vi "Main.vi"() -> ()   [LabVIEW 2020, in "Ex 1 - Simulated LP.lvlib"]
uses:
  Ex 1 - Simulated LP.lvlib
  <vilib>/measure/macond.llb/IIR Filter for 1 Chan.vi
  <vilib>/measure/matone.llb/Extract Single Tone Information 1 Chan.vi
  <vilib>/measure/NI_MABase.lvlib
  <vilib>/measure/NI_MAPro.lvlib
panel:
  in  "Title":string="BODE PLOT (FH Joanneum)"
  in  "Cut-off Frequency":dbl=100000.0 format="%#_6p"
  in  "Order":i32=2
  in  "Topology":T1(ring)=enum."Butterworth"
  in  "Start":bool
  in  "Timing (ms)":u32
  in  "stop":bool
  in  "Amplitude":dbl=10.0
  in  "Freq. Step":dbl=1000.0 caption="Frequency Step" format="%#_6p"
  in  "Stop Frequ.":dbl=1000000.0 caption="Stop Frequency" format="%#_6p"
  in  "Start Freq.":dbl=1000.0 caption="Start Frequency" format="%#_6p"
  out "Waveform Graph":waveform(dbl)[](graph)
  out "Magnitude":cluster{"X":dbl, "Y":dbl}[](graph)=[{"X"=1000.0, "Y"=0.0}, {"X"=2000.0, "Y"=0.0}, {"X"=3000.0, "Y"=-4.7058926481545906e-07}, {"X"=4000.0, "Y"=-4.235994406084898e-06}, {"X"=5000.0, "Y"=-1.5203059229301419e-05}, {"X"=6000.0, "Y"=-3.8126734506028564e-05}, {"X"=7000.0, "Y"=-7.876650446461324e-05}, {"X"=8000.0, "Y"=-0.0001439147572122518}, {"X"=9000.0, "Y"=-0.00024140357010209228}, {"X"=10000.0, "Y"=-0.00038010648213580877}, {"X"=11000.0, "Y"=-0.0005699385936490564}, {"X"=12000.0, "Y"=-0.0008218558292255898}, {"X"=13000.0, "Y"=-0.0011478535749765322}, {"X"=14000.0, "Y"=-0.001560964706777549}, {"X"=15000.0, "Y"=-0.0020752569545813126}, {"X"=16000.0, "Y"=-0.0027058295134445385}, {"X"=17000.0, "Y"=-0.003468808794544552}, {"X"=18000.0, "Y"=-0.004381343195914282}, {"X"=19000.0, "Y"=-0.005461596762600354}, {"X"=20000.0, "Y"=-0.006728741598133291}, {"X"=21000.0, "Y"=-0.008202948881267663}, {"X"=22000.0, "Y"=-0.009905378335483283}, {"X"=23000.0, "Y"=-0.011858165993133746}, {"X"=24000.0, "Y"=-0.01408441009127886}, {"X"=25000.0, "Y"=-0.016608154932204067}, {"X"=26000.0, "Y"=-0.019454372539159805}, {"X"=27000.0, "Y"=-0.022648941935728285}, {"X"=28000.0, "Y"=-0.026218625878250468}, {"X"=29000.0, "Y"=-0.030191044870233313}, {"X"=30000.0, "Y"=-0.03459464829307458}, {"X"=31000.0, "Y"=-0.0394586824895382}, {"X"=32000.0, "Y"=-0.04481315564715423}, {"X"=33000.0, "Y"=-0.05068879933203461}, {"X"=34000.0, "Y"=-0.05711702654319666}, {"X"=35000.0, "Y"=-0.06412988616203336}, {"X"=36000.0, "Y"=-0.07176001369565913}, {"X"=37000.0, "Y"=-0.0800405782282296}, {"X"=38000.0, "Y"=-0.08900522551567218}, {"X"=39000.0, "Y"=-0.09868801718765945}, {"X"=40000.0, "Y"=-0.10912336604225487}, {"X"=41000.0, "Y"=-0.12034596745431009}, {"X"=42000.0, "Y"=-0.1323907269484053}, {"X"=43000.0, "Y"=-0.14529268402125897}, {"X"=44000.0, "Y"=-0.15908693233963056}, {"X"=45000.0, "Y"=-0.1738085364745352}, {"X"=46000.0, "Y"=-0.18949244537640458}, {"X"=47000.0, "Y"=-0.20617340283688407}, {"X"=48000.0, "Y"=-0.223885855226176}, {"X"=49000.0, "Y"=-0.24266385683539424}, {"X"=50000.0, "Y"=-0.26254097319813513}, {"X"=51000.0, "Y"=-0.2835501828093141}, {"X"=52000.0, "Y"=-0.305723777689094}, {"X"=53000.0, "Y"=-0.3290932632891572}, {"X"=54000.0, "Y"=-0.3536892700554042}, {"X"=55000.0, "Y"=-0.37954141196215424}, {"X"=56000.0, "Y"=-0.4066782422305516}, {"X"=57000.0, "Y"=-0.4351271247729583}, {"X"=58000.0, "Y"=-0.46491414587534396}, {"X"=59000.0, "Y"=-0.49606402204891537}, {"X"=60000.0, "Y"=-0.5286000113418585}, {"X"=61000.0, "Y"=-0.5625438287314889}, {"X"=62000.0, "Y"=-0.5979155661973111}, {"X"=63000.0, "Y"=-0.6347336180540024}, {"X"=64000.0, "Y"=-0.6730146121003455}, {"X"=65000.0, "Y"=-0.7127733470961873}, {"X"=66000.0, "Y"=-0.7540227370395547}, {"X"=67000.0, "Y"=-0.7967737626708788}, {"X"=68000.0, "Y"=-0.8410354305647758}, {"X"=69000.0, "Y"=-0.8868147401211939}, {"X"=70000.0, "Y"=-0.9341166586949998}, {"X"=71000.0, "Y"=-0.9829441050379926}, {"X"=72000.0, "Y"=-1.0332979411576286}, {"X"=73000.0, "Y"=-1.085176972621999}, {"X"=74000.0, "Y"=-1.1385779572743775}, {"X"=75000.0, "Y"=-1.1934956222444086}, {"X"=76000.0, "Y"=-1.2499226890777513}, {"X"=77000.0, "Y"=-1.307849906737507}, {"X"=78000.0, "Y"=-1.367266092175559}, {"X"=79000.0, "Y"=-1.4281581781011314}, {"X"=80000.0, "Y"=-1.490511267540837}, {"X"=81000.0, "Y"=-1.5543086947183857}, {"X"=82000.0, "Y"=-1.619532091760238}, {"X"=83000.0, "Y"=-1.6861614606881672}, {"X"=84000.0, "Y"=-1.7541752501398347}, {"X"=85000.0, "Y"=-1.8235504362403714}, {"X"=86000.0, "Y"=-1.894262607028815}, {"X"=87000.0, "Y"=-1.9662860498489467}, {"X"=88000.0, "Y"=-2.039593841103528}, {"X"=89000.0, "Y"=-2.1141579377887303}, {"X"=90000.0, "Y"=-2.189949270229024}, {"X"=91000.0, "Y"=-2.2669378354594665}, {"X"=92000.0, "Y"=-2.345092790717058}, {"X"=93000.0, "Y"=-2.424382546535789}, {"X"=94000.0, "Y"=-2.504774858965561}, {"X"=95000.0, "Y"=-2.586236920475759}, {"X"=96000.0, "Y"=-2.668735449101548}, {"X"=97000.0, "Y"=-2.752236775525848}, {"X"=98000.0, "Y"=-2.8367069276892405}, {"X"=99000.0, "Y"=-2.922111712666817}, {"X"=100000.0, "Y"=-3.008416795542534}, {"X"=101000.0, "Y"=-3.0955877750590197}, {"X"=102000.0, "Y"=-3.18359025585552}, {"X"=103000.0, "Y"=-3.272389917143707}, {"X"=104000.0, "Y"=-3.3619525777045487}, {"X"=105000.0, "Y"=-3.452244257121428}, {"X"=106000.0, "Y"=-3.5432312331963423}, {"X"=107000.0, "Y"=-3.634880095522957}, {"X"=108000.0, "Y"=-3.7271577952177553}, {"X"=109000.0, "Y"=-3.820031690834062}, {"X"=110000.0, "Y"=-3.913469590505059}, {"X"=111000.0, "Y"=-4.007439790382403}, {"X"=112000.0, "Y"=-4.101911109452055}, {"X"=113000.0, "Y"=-4.196852920828556}, {"X"=114000.0, "Y"=-4.292235179634819}, {"X"=115000.0, "Y"=-4.3880284475928875}, {"X"=116000.0, "Y"=-4.484203914453854}, {"X"=117000.0, "Y"=-4.580733416407038}, {"X"=118000.0, "Y"=-4.677589451610474}, {"X"=119000.0, "Y"=-4.774745192989594}, {"X"=120000.0, "Y"=-4.872174498456132}, {"X"=121000.0, "Y"=-4.96985191869544}, {"X"=122000.0, "Y"=-5.067752702673315}, {"X"=123000.0, "Y"=-5.165855460663462}, {"X"=124000.0, "Y"=-5.2641319673999405}, {"X"=125000.0, "Y"=-5.362561822358578}, {"X"=126000.0, "Y"=-5.461123081246283}, {"X"=127000.0, "Y"=-5.5597944964429304}, {"X"=128000.0, "Y"=-5.658555511891694}, {"X"=129000.0, "Y"=-5.757386256696502}, {"X"=130000.0, "Y"=-5.8562675375405355}, {"X"=131000.0, "Y"=-5.955180830049295}, {"X"=132000.0, "Y"=-6.0541082692101345}, {"X"=133000.0, "Y"=-6.1530326389465}, {"X"=134000.0, "Y"=-6.251937360956765}, {"X"=135000.0, "Y"=-6.3508064829043125}, {"X"=136000.0, "Y"=-6.449624666050838}, {"X"=137000.0, "Y"=-6.548377172415963}, {"X"=138000.0, "Y"=-6.64704985153692}, {"X"=139000.0, "Y"=-6.745629126905376}, {"X"=140000.0, "Y"=-6.844101982144563}, {"X"=141000.0, "Y"=-6.942455946989798}, {"X"=142000.0, "Y"=-7.040679083126048}, {"X"=143000.0, "Y"=-7.138759969940191}, {"X"=144000.0, "Y"=-7.236687690232017}, {"X"=145000.0, "Y"=-7.334451815927893}, {"X"=146000.0, "Y"=-7.432042393834642}, {"X"=147000.0, "Y"=-7.529449931475854}, {"X"=148000.0, "Y"=-7.626665383033114}, {"X"=149000.0, "Y"=-7.723680135429653}, {"X"=150000.0, "Y"=-7.820485994576546}, {"X"=151000.0, "Y"=-7.917075171808563}, {"X"=152000.0, "Y"=-8.013440270519457}, {"X"=153000.0, "Y"=-8.109574273030688}, {"X"=154000.0, "Y"=-8.205470527694786}, {"X"=155000.0, "Y"=-8.301122736248846}, {"X"=156000.0, "Y"=-8.39652494143235}, {"X"=157000.0, "Y"=-8.491671514879934}, {"X"=158000.0, "Y"=-8.586557145285052}, {"X"=159000.0, "Y"=-8.681176826856413}, {"X"=160000.0, "Y"=-8.775525848057779}, {"X"=161000.0, "Y"=-8.869599780639252}, {"X"=162000.0, "Y"=-8.963394468965031}, {"X"=163000.0, "Y"=-9.05690601963175}, {"X"=164000.0, "Y"=-9.150130791383427}, {"X"=165000.0, "Y"=-9.24306538531414}, {"X"=166000.0, "Y"=-9.335706635368732}, {"X"=167000.0, "Y"=-9.42805159912396}, {"X"=168000.0, "Y"=-9.520097548858109}, {"X"=169000.0, "Y"=-9.611841962904887}, {"X"=170000.0, "Y"=-9.703282517275158}, {"X"=171000.0, "Y"=-9.794417077563297}, {"X"=172000.0, "Y"=-9.885243691108869}, {"X"=173000.0, "Y"=-9.975760579431988}, {"X"=174000.0, "Y"=-10.065966130914283}, {"X"=175000.0, "Y"=-10.155858893742307}, {"X"=176000.0, "Y"=-10.245437569088836}, {"X"=177000.0, "Y"=-10.334701004534255}, {"X"=178000.0, "Y"=-10.423648187726064}, {"X"=179000.0, "Y"=-10.512278240262589}, {"X"=180000.0, "Y"=-10.600590411796667}, {"X"=181000.0, "Y"=-10.688584074359479}, {"X"=182000.0, "Y"=-10.776258716886478}, {"X"=183000.0, "Y"=-10.863613939954625}, {"X"=184000.0, "Y"=-10.950649450707068}, {"X"=185000.0, "Y"=-11.037365057981665}, {"X"=186000.0, "Y"=-11.123760667607058}, {"X"=187000.0, "Y"=-11.209836277898013}, {"X"=188000.0, "Y"=-11.295591975305555}, {"X"=189000.0, "Y"=-11.381027930247125}, {"X"=190000.0, "Y"=-11.466144393097576}, {"X"=191000.0, "Y"=-11.55094169032801}, {"X"=192000.0, "Y"=-11.635420220809047}, {"X"=193000.0, "Y"=-11.719580452252224}, {"X"=194000.0, "Y"=-11.803422917791085}, {"X"=195000.0, "Y"=-11.886948212708035}, {"X"=196000.0, "Y"=-11.970156991279863}, {"X"=197000.0, "Y"=-12.053049963763204}, {"X"=198000.0, "Y"=-12.135627893489993}, {"X"=199000.0, "Y"=-12.217891594089759}, {"X"=200000.0, "Y"=-12.29984192682171}, {"X"=201000.0, "Y"=-12.381479798015718}, {"X"=202000.0, "Y"=-12.46280615661728}, {"X"=203000.0, "Y"=-12.543821991840698}, {"X"=204000.0, "Y"=-12.62452833091158}, {"X"=205000.0, "Y"=-12.70492623690393}, {"X"=206000.0, "Y"=-12.78501680667606}, {"X"=207000.0, "Y"=-12.864801168882458}, {"X"=208000.0, "Y"=-12.944280482076318}, {"X"=209000.0, "Y"=-13.023455932887927}, {"X"=210000.0, "Y"=-13.102328734286502}, {"X"=211000.0, "Y"=-13.180900123907104}, {"X"=212000.0, "Y"=-13.25917136245713}, {"X"=213000.0, "Y"=-13.337143732188219}, {"X"=214000.0, "Y"=-13.414818535431191}, {"X"=215000.0, "Y"=-13.492197093200705}, {"X"=216000.0, "Y"=-13.569280743854248}, {"X"=217000.0, "Y"=-13.646070841812053}, {"X"=218000.0, "Y"=-13.72256875633643}, {"X"=219000.0, "Y"=-13.798775870356472}, {"X"=220000.0, "Y"=-13.8746935793548}, {"X"=221000.0, "Y"=-13.950323290295861}, {"X"=222000.0, "Y"=-14.025666420605168}, {"X"=223000.0, "Y"=-14.100724397194575}, {"X"=224000.0, "Y"=-14.17549865552884}, {"X"=225000.0, "Y"=-14.24999063874024}, {"X"=226000.0, "Y"=-14.324201796771556}, {"X"=227000.0, "Y"=-14.398133585574461}, {"X"=228000.0, "Y"=-14.471787466329765}, {"X"=229000.0, "Y"=-14.545164904715811}, {"X"=230000.0, "Y"=-14.618267370197653}, {"X"=231000.0, "Y"=-14.691096335362255}, {"X"=232000.0, "Y"=-14.763653275275736}, {"X"=233000.0, "Y"=-14.835939666878035}, {"X"=234000.0, "Y"=-14.907956988400237}, {"X"=235000.0, "Y"=-14.979706718812793}, {"X"=236000.0, "Y"=-15.05119033729854}, {"X"=237000.0, "Y"=-15.122409322755534}, {"X"=238000.0, "Y"=-15.193365153317533}, {"X"=239000.0, "Y"=-15.264059305905214}, {"X"=240000.0, "Y"=-15.334493255794165}, {"X"=241000.0, "Y"=-15.404668476206185}, {"X"=242000.0, "Y"=-15.474586437922506}, {"X"=243000.0, "Y"=-15.544248608915323}, {"X"=244000.0, "Y"=-15.61365645399822}, {"X"=245000.0, "Y"=-15.682811434497662}, {"X"=246000.0, "Y"=-15.751715007934507}, {"X"=247000.0, "Y"=-15.820368627733375}, {"X"=248000.0, "Y"=-15.888773742935978}, {"X"=249000.0, "Y"=-15.956931797937868}, {"X"=250000.0, "Y"=-16.024844232238152}, {"X"=251000.0, "Y"=-16.0925124802025}, {"X"=252000.0, "Y"=-16.15993797083511}, {"X"=253000.0, "Y"=-16.227122127574578}, {"X"=254000.0, "Y"=-16.294066368090544}, {"X"=255000.0, "Y"=-16.360772104096878}, {"X"=256000.0, "Y"=-16.42724074118115}, {"X"=257000.0, "Y"=-16.493473678633453}, {"X"=258000.0, "Y"=-16.559472309295167}, {"X"=259000.0, "Y"=-16.625238019415402}, {"X"=260000.0, "Y"=-16.690772188512703}, {"X"=261000.0, "Y"=-16.756076189253196}, {"X"=262000.0, "Y"=-16.82115138732697}, {"X"=263000.0, "Y"=-16.885999141346083}, {"X"=264000.0, "Y"=-16.950620802738797}, {"X"=265000.0, "Y"=-17.015017715654785}, {"X"=266000.0, "Y"=-17.079191216883608}, {"X"=267000.0, "Y"=-17.143142635769106}, {"X"=268000.0, "Y"=-17.206873294141282}, {"X"=269000.0, "Y"=-17.270384506246447}, {"X"=270000.0, "Y"=-17.33367757868715}, {"X"=271000.0, "Y"=-17.396753810367407}, {"X"=272000.0, "Y"=-17.45961449244436}, {"X"=273000.0, "Y"=-17.522260908281318}, {"X"=274000.0, "Y"=-17.58469433341141}, {"X"=275000.0, "Y"=-17.646916035498602}, {"X"=276000.0, "Y"=-17.708927274314817}, {"X"=277000.0, "Y"=-17.770729301707398}, {"X"=278000.0, "Y"=-17.832323361580443}, {"X"=279000.0, "Y"=-17.893710689877405}, {"X"=280000.0, "Y"=-17.954892514566296}, {"X"=281000.0, "Y"=-18.01587005563178}, {"X"=282000.0, "Y"=-18.07664452506634}, {"X"=283000.0, "Y"=-18.137217126865238}, {"X"=284000.0, "Y"=-18.197589057027997}, {"X"=285000.0, "Y"=-18.257761503562023}, {"X"=286000.0, "Y"=-18.31773564648534}, {"X"=287000.0, "Y"=-18.377512657836736}, {"X"=288000.0, "Y"=-18.43709370168274}, {"X"=289000.0, "Y"=-18.496479934135166}, {"X"=290000.0, "Y"=-18.555672503361244}, {"X"=291000.0, "Y"=-18.614672549604855}, {"X"=292000.0, "Y"=-18.673481205205256}, {"X"=293000.0, "Y"=-18.73209959461389}, {"X"=294000.0, "Y"=-18.79052883442349}, {"X"=295000.0, "Y"=-18.848770033390608}, {"X"=296000.0, "Y"=-18.90682429245923}, {"X"=297000.0, "Y"=-18.964692704793407}, {"X"=298000.0, "Y"=-19.02237635580446}, {"X"=299000.0, "Y"=-19.079876323179942}, {"X"=300000.0, "Y"=-19.137193676920692}, {"X"=301000.0, "Y"=-19.194329479368367}, {"X"=302000.0, "Y"=-19.25128478524589}, {"X"=303000.0, "Y"=-19.30806064168852}, {"X"=304000.0, "Y"=-19.36465808828178}, {"X"=305000.0, "Y"=-19.42107815710046}, {"X"=306000.0, "Y"=-19.477321872746593}, {"X"=307000.0, "Y"=-19.533390252386738}, {"X"=308000.0, "Y"=-19.589284305794557}, {"X"=309000.0, "Y"=-19.645005035390913}, {"X"=310000.0, "Y"=-19.70055343628699}, {"X"=311000.0, "Y"=-19.75593049632279}, {"X"=312000.0, "Y"=-19.811137196111925}, {"X"=313000.0, "Y"=-19.86617450908731}, {"X"=314000.0, "Y"=-19.921043401540246}, {"X"=315000.0, "Y"=-19.975744832667978}, {"X"=316000.0, "Y"=-20.03027975461794}, {"X"=317000.0, "Y"=-20.084649112531817}, {"X"=318000.0, "Y"=-20.13885384459283}, {"X"=319000.0, "Y"=-20.192894882068188}, {"X"=320000.0, "Y"=-20.24677314935738}, {"X"=321000.0, "Y"=-20.30048956403927}, {"X"=322000.0, "Y"=-20.35404503691563}, {"X"=323000.0, "Y"=-20.407440472061595}, {"X"=324000.0, "Y"=-20.46067676686917}, {"X"=325000.0, "Y"=-20.513754812092763}, {"X"=326000.0, "Y"=-20.566675491902643}, {"X"=327000.0, "Y"=-20.619439683925968}, {"X"=328000.0, "Y"=-20.672048259297352}, {"X"=329000.0, "Y"=-20.724502082703424}, {"X"=330000.0, "Y"=-20.77680201243293}, {"X"=331000.0, "Y"=-20.828948900420343}, {"X"=332000.0, "Y"=-20.880943592297548}, {"X"=333000.0, "Y"=-20.932786927438933}, {"X"=334000.0, "Y"=-20.9844797390068}, {"X"=335000.0, "Y"=-21.036022853999793}, {"X"=336000.0, "Y"=-21.08741709330269}, {"X"=337000.0, "Y"=-21.138663271728486}, {"X"=338000.0, "Y"=-21.189762198067818}, {"X"=339000.0, "Y"=-21.240714675137014}, {"X"=340000.0, "Y"=-21.29152149982074}, {"X"=341000.0, "Y"=-21.342183463123405}, {"X"=342000.0, "Y"=-21.392701350207087}, {"X"=343000.0, "Y"=-21.44307594045021}, {"X"=344000.0, "Y"=-21.493308007482206}, {"X"=345000.0, "Y"=-21.543398319233695}, {"X"=346000.0, "Y"=-21.59334763798313}, {"X"=347000.0, "Y"=-21.643156720399933}, {"X"=348000.0, "Y"=-21.692826317589663}, {"X"=349000.0, "Y"=-21.742357175140654}, {"X"=350000.0, "Y"=-21.791750033167908}, {"X"=351000.0, "Y"=-21.84100562635718}, {"X"=352000.0, "Y"=-21.89012468401001}, {"X"=353000.0, "Y"=-21.939107930083615}, {"X"=354000.0, "Y"=-21.987956083242338}, {"X"=355000.0, "Y"=-22.036669856894306}, {"X"=356000.0, "Y"=-22.085249959237782}, {"X"=357000.0, "Y"=-22.133697093305603}, {"X"=358000.0, "Y"=-22.18201195700206}, {"X"=359000.0, "Y"=-22.23019524314994}, {"X"=360000.0, "Y"=-22.278247639534484}, {"X"=361000.0, "Y"=-22.326169828940024}, {"X"=362000.0, "Y"=-22.37396248919461}, {"X"=363000.0, "Y"=-22.42162629321072}, {"X"=364000.0, "Y"=-22.46916190902627}, {"X"=365000.0, "Y"=-22.51656999984677}, {"X"=366000.0, "Y"=-22.563851224082892}, {"X"=367000.0, "Y"=-22.61100623539201}, {"X"=368000.0, "Y"=-22.658035682721156}, {"X"=369000.0, "Y"=-22.70494021034019}, {"X"=370000.0, "Y"=-22.751720457886616}, {"X"=371000.0, "Y"=-22.798377060403567}, {"X"=372000.0, "Y"=-22.844910648375144}, {"X"=373000.0, "Y"=-22.89132184776854}, {"X"=374000.0, "Y"=-22.93761128007275}, {"X"=375000.0, "Y"=-22.98377956233007}, {"X"=376000.0, "Y"=-23.02982730718344}, {"X"=377000.0, "Y"=-23.075755122905733}, {"X"=378000.0, "Y"=-23.121563613438134}, {"X"=379000.0, "Y"=-23.167253378429805}, {"X"=380000.0, "Y"=-23.212825013272816}, {"X"=381000.0, "Y"=-23.25827910913671}, {"X"=382000.0, "Y"=-23.303616253006396}, {"X"=383000.0, "Y"=-23.348837027716044}, {"X"=384000.0, "Y"=-23.393942011982563}, {"X"=385000.0, "Y"=-23.438931780447795}, {"X"=386000.0, "Y"=-23.483806903704433}, {"X"=387000.0, "Y"=-23.528567948333343}, {"X"=388000.0, "Y"=-23.573215476941588}, {"X"=389000.0, "Y"=-23.617750048189144}, {"X"=390000.0, "Y"=-23.66217221682743}, {"X"=391000.0, "Y"=-23.706482533733094}, {"X"=392000.0, "Y"=-23.750681545933332}, {"X"=393000.0, "Y"=-23.794769796649867}, {"X"=394000.0, "Y"=-23.838747825321406}, {"X"=395000.0, "Y"=-23.88261616764083}, {"X"=396000.0, "Y"=-23.926375355584124}, {"X"=397000.0, "Y"=-23.970025917445227}, {"X"=398000.0, "Y"=-24.013568377865187}, {"X"=399000.0, "Y"=-24.057003257860572}, {"X"=400000.0, "Y"=-24.10033107486025}, {"X"=401000.0, "Y"=-24.143552342728164}, {"X"=402000.0, "Y"=-24.186667571800925}, {"X"=403000.0, "Y"=-24.229677268912635}, {"X"=404000.0, "Y"=-24.27258193742547}, {"X"=405000.0, "Y"=-24.31538207725987}, {"X"=406000.0, "Y"=-24.358078184921773}, {"X"=407000.0, "Y"=-24.400670753535884}, {"X"=408000.0, "Y"=-24.44316027286812}, {"X"=409000.0, "Y"=-24.485547229356857}, {"X"=410000.0, "Y"=-24.52783210614127}, {"X"=411000.0, "Y"=-24.570015383089196}, {"X"=412000.0, "Y"=-24.61209753682173}, {"X"=413000.0, "Y"=-24.654079040745653}, {"X"=414000.0, "Y"=-24.695960365074168}, {"X"=415000.0, "Y"=-24.737741976860864}, {"X"=416000.0, "Y"=-24.77942434001666}, {"X"=417000.0, "Y"=-24.82100791534731}, {"X"=418000.0, "Y"=-24.86249316056935}, {"X"=419000.0, "Y"=-24.90388053034212}, {"X"=420000.0, "Y"=-24.94517047629154}, {"X"=421000.0, "Y"=-24.986363447033124}, {"X"=422000.0, "Y"=-25.027459888200625}, {"X"=423000.0, "Y"=-25.068460242470273}, {"X"=424000.0, "Y"=-25.109364949581167}, {"X"=425000.0, "Y"=-25.150174446366456}, {"X"=426000.0, "Y"=-25.190889166771534}, {"X"=427000.0, "Y"=-25.231509541879596}, {"X"=428000.0, "Y"=-25.272035999939504}, {"X"=429000.0, "Y"=-25.3124689663831}, {"X"=430000.0, "Y"=-25.352808863849074}, {"X"=431000.0, "Y"=-25.393056112212694}, {"X"=432000.0, "Y"=-25.4332111286003}, {"X"=433000.0, "Y"=-25.47327432741703}, {"X"=434000.0, "Y"=-25.513246120368187}, {"X"=435000.0, "Y"=-25.55312691647895}, {"X"=436000.0, "Y"=-25.592917122120433}, {"X"=437000.0, "Y"=-25.63261714102832}, {"X"=438000.0, "Y"=-25.672227374327004}, {"X"=439000.0, "Y"=-25.711748220546365}, {"X"=440000.0, "Y"=-25.75118007564892}, {"X"=441000.0, "Y"=-25.79052333304562}, {"X"=442000.0, "Y"=-25.82977838362134}, {"X"=443000.0, "Y"=-25.868945615751024}, {"X"=444000.0, "Y"=-25.908025415322523}, {"X"=445000.0, "Y"=-25.94701816575757}, {"X"=446000.0, "Y"=-25.985924248029768}, {"X"=447000.0, "Y"=-26.02474404068348}, {"X"=448000.0, "Y"=-26.0634779198569}, {"X"=449000.0, "Y"=-26.102126259299865}, {"X"=450000.0, "Y"=-26.140689430392534}, {"X"=451000.0, "Y"=-26.179167802165793}, {"X"=452000.0, "Y"=-26.21756174131789}, {"X"=453000.0, "Y"=-26.2558716122367}, {"X"=454000.0, "Y"=-26.294097777014677}, {"X"=455000.0, "Y"=-26.332240595468672}, {"X"=456000.0, "Y"=-26.370300425159265}, {"X"=457000.0, "Y"=-26.408277621408175}, {"X"=458000.0, "Y"=-26.44617253731315}, {"X"=459000.0, "Y"=-26.48398552377118}, {"X"=460000.0, "Y"=-26.521716929493103}, {"X"=461000.0, "Y"=-26.55936710101871}, {"X"=462000.0, "Y"=-26.596936382740356}, {"X"=463000.0, "Y"=-26.634425116910347}, {"X"=464000.0, "Y"=-26.67183364367007}, {"X"=465000.0, "Y"=-26.709162301053972}, {"X"=466000.0, "Y"=-26.746411425019033}, {"X"=467000.0, "Y"=-26.783581349447193}, {"X"=468000.0, "Y"=-26.820672406176076}, {"X"=469000.0, "Y"=-26.857684925002296}, {"X"=470000.0, "Y"=-26.894619233706013}, {"X"=471000.0, "Y"=-26.931475658065196}, {"X"=472000.0, "Y"=-26.968254521867316}, {"X"=473000.0, "Y"=-27.00495614692938}, {"X"=474000.0, "Y"=-27.04158085311196}, {"X"=475000.0, "Y"=-27.078128958332513}, {"X"=476000.0, "Y"=-27.11460077858323}, {"X"=477000.0, "Y"=-27.15099662794558}, {"X"=478000.0, "Y"=-27.18731681860362}, {"X"=479000.0, "Y"=-27.223561660859108}, {"X"=480000.0, "Y"=-27.25973146314875}, {"X"=481000.0, "Y"=-27.295826532053105}, {"X"=482000.0, "Y"=-27.331847172318355}, {"X"=483000.0, "Y"=-27.367793686861894}, {"X"=484000.0, "Y"=-27.403666376796206}, {"X"=485000.0, "Y"=-27.43946554143227}, {"X"=486000.0, "Y"=-27.475191478301504}, {"X"=487000.0, "Y"=-27.510844483167425}, {"X"=488000.0, "Y"=-27.54642485003413}, {"X"=489000.0, "Y"=-27.581932871167577}, {"X"=490000.0, "Y"=-27.617368837105452}, {"X"=491000.0, "Y"=-27.652733036667758}, {"X"=492000.0, "Y"=-27.6880257569723}, {"X"=493000.0, "Y"=-27.723247283449535}, {"X"=494000.0, "Y"=-27.758397899852273}, {"X"=495000.0, "Y"=-27.79347788826907}, {"X"=496000.0, "Y"=-27.828487529137384}, {"X"=497000.0, "Y"=-27.863427101255837}, {"X"=498000.0, "Y"=-27.898296881798885}, {"X"=499000.0, "Y"=-27.933097146324034}, {"X"=500000.0, "Y"=-27.967828168787964}, {"X"=501000.0, "Y"=-28.002490221556535}, {"X"=502000.0, "Y"=-28.037083575420617}, {"X"=503000.0, "Y"=-28.07160849959924}, {"X"=504000.0, "Y"=-28.10606526176319}, {"X"=505000.0, "Y"=-28.140454128037284}, {"X"=506000.0, "Y"=-28.174775363014376}, {"X"=507000.0, "Y"=-28.209029229769857}, {"X"=508000.0, "Y"=-28.243215989867952}, {"X"=509000.0, "Y"=-28.277335903376585}, {"X"=510000.0, "Y"=-28.31138922887826}, {"X"=511000.0, "Y"=-28.34537622347772}, {"X"=512000.0, "Y"=-28.379297142819375}, {"X"=513000.0, "Y"=-28.413152241089268}, {"X"=514000.0, "Y"=-28.446941771034687}, {"X"=515000.0, "Y"=-28.48066598396677}, {"X"=516000.0, "Y"=-28.514325129778868}, {"X"=517000.0, "Y"=-28.547919456951803}, {"X"=518000.0, "Y"=-28.581449212563026}, {"X"=519000.0, "Y"=-28.6149146423022}, {"X"=520000.0, "Y"=-28.648315990477467}, {"X"=521000.0, "Y"=-28.68165350002615}, {"X"=522000.0, "Y"=-28.714927412527476}, {"X"=523000.0, "Y"=-28.74813796820463}, {"X"=524000.0, "Y"=-28.78128540594725}, {"X"=525000.0, "Y"=-28.814369963307882}, {"X"=526000.0, "Y"=-28.847391876520156}, {"X"=527000.0, "Y"=-28.88035138050837}, {"X"=528000.0, "Y"=-28.91324870888827}, {"X"=529000.0, "Y"=-28.946084093988848}, {"X"=530000.0, "Y"=-28.97885776685227}, {"X"=531000.0, "Y"=-29.011569957245577}, {"X"=532000.0, "Y"=-29.044220893674435}, {"X"=533000.0, "Y"=-29.076810803383207}, {"X"=534000.0, "Y"=-29.10933991237328}, {"X"=535000.0, "Y"=-29.141808445405026}, {"X"=536000.0, "Y"=-29.174216626010733}, {"X"=537000.0, "Y"=-29.20656467650066}, {"X"=538000.0, "Y"=-29.238852817976007}, {"X"=539000.0, "Y"=-29.27108127033096}, {"X"=540000.0, "Y"=-29.30325025226701}, {"X"=541000.0, "Y"=-29.335359981297003}, {"X"=542000.0, "Y"=-29.36741067376016}, {"X"=543000.0, "Y"=-29.39940254482184}, {"X"=544000.0, "Y"=-29.431335808486594}, {"X"=545000.0, "Y"=-29.463210677608487}, {"X"=546000.0, "Y"=-29.495027363893907}, {"X"=547000.0, "Y"=-29.526786077910756}, {"X"=548000.0, "Y"=-29.558487029102395}, {"X"=549000.0, "Y"=-29.59013042578624}, {"X"=550000.0, "Y"=-29.62171647516972}, {"X"=551000.0, "Y"=-29.65324538335203}, {"X"=552000.0, "Y"=-29.684717355337288}, {"X"=553000.0, "Y"=-29.71613259503559}, {"X"=554000.0, "Y"=-29.747491305277876}, {"X"=555000.0, "Y"=-29.778793687818563}, {"X"=556000.0, "Y"=-29.810039943343412}, {"X"=557000.0, "Y"=-29.841230271479375}, {"X"=558000.0, "Y"=-29.872364870799988}, {"X"=559000.0, "Y"=-29.903443938831682}, {"X"=560000.0, "Y"=-29.934467672063576}, {"X"=561000.0, "Y"=-29.965436265953052}, {"X"=562000.0, "Y"=-29.996349914934473}, {"X"=563000.0, "Y"=-30.02720881242214}, {"X"=564000.0, "Y"=-30.05801315082287}, {"X"=565000.0, "Y"=-30.08876312153804}, {"X"=566000.0, "Y"=-30.11945891497295}, {"X"=567000.0, "Y"=-30.15010072054388}, {"X"=568000.0, "Y"=-30.180688726683023}, {"X"=569000.0, "Y"=-30.21122312084708}, {"X"=570000.0, "Y"=-30.2417040895224}, {"X"=571000.0, "Y"=-30.272131818232452}, {"X"=572000.0, "Y"=-30.30250649154473}, {"X"=573000.0, "Y"=-30.332828293074083}, {"X"=574000.0, "Y"=-30.363097405495566}, {"X"=575000.0, "Y"=-30.393314010542984}, {"X"=576000.0, "Y"=-30.42347828902068}, {"X"=577000.0, "Y"=-30.453590420810226}, {"X"=578000.0, "Y"=-30.483650584869967}, {"X"=579000.0, "Y"=-30.513658959249614}, {"X"=580000.0, "Y"=-30.543615721091676}, {"X"=581000.0, "Y"=-30.573521046636394}, {"X"=582000.0, "Y"=-30.603375111232186}, {"X"=583000.0, "Y"=-30.633178089339438}, {"X"=584000.0, "Y"=-30.66293015453121}, {"X"=585000.0, "Y"=-30.692631479511586}, {"X"=586000.0, "Y"=-30.72228223610688}, {"X"=587000.0, "Y"=-30.751882595283075}, {"X"=588000.0, "Y"=-30.781432727143653}, {"X"=589000.0, "Y"=-30.810932800942158}, {"X"=590000.0, "Y"=-30.84038298508052}, {"X"=591000.0, "Y"=-30.86978344712017}, {"X"=592000.0, "Y"=-30.899134353785023}, {"X"=593000.0, "Y"=-30.92843587096842}, {"X"=594000.0, "Y"=-30.957688163736847}, {"X"=595000.0, "Y"=-30.986891396336773}, {"X"=596000.0, "Y"=-31.01604573220037}, {"X"=597000.0, "Y"=-31.045151333947977}, {"X"=598000.0, "Y"=-31.07420836339722}, {"X"=599000.0, "Y"=-31.103216981565463}, {"X"=600000.0, "Y"=-31.132177348675818}, {"X"=601000.0, "Y"=-31.161089624164823}, {"X"=602000.0, "Y"=-31.189953966680875}, {"X"=603000.0, "Y"=-31.218770534096414}, {"X"=604000.0, "Y"=-31.247539483511723}, {"X"=605000.0, "Y"=-31.276260971254196}, {"X"=606000.0, "Y"=-31.30493515289028}, {"X"=607000.0, "Y"=-31.3335621832276}, {"X"=608000.0, "Y"=-31.362142216318286}, {"X"=609000.0, "Y"=-31.390675405466514}, {"X"=610000.0, "Y"=-31.41916190323192}, {"X"=611000.0, "Y"=-31.447601861433547}, {"X"=612000.0, "Y"=-31.475995431157024}, {"X"=613000.0, "Y"=-31.504342762757467}, {"X"=614000.0, "Y"=-31.53264400586273}, {"X"=615000.0, "Y"=-31.56089930938493}, {"X"=616000.0, "Y"=-31.58910882151202}, {"X"=617000.0, "Y"=-31.6172726897264}, {"X"=618000.0, "Y"=-31.645391060800495}, {"X"=619000.0, "Y"=-31.67346408080511}, {"X"=620000.0, "Y"=-31.701491895111964}, {"X"=621000.0, "Y"=-31.72947464839925}, {"X"=622000.0, "Y"=-31.757412484655276}, {"X"=623000.0, "Y"=-31.78530554718258}, {"X"=624000.0, "Y"=-31.81315397860447}, {"X"=625000.0, "Y"=-31.84095792086582}, {"X"=626000.0, "Y"=-31.868717515241364}, {"X"=627000.0, "Y"=-31.896432902333757}, {"X"=628000.0, "Y"=-31.924104222085955}, {"X"=629000.0, "Y"=-31.95173161377712}, {"X"=630000.0, "Y"=-31.979315216035424}, {"X"=631000.0, "Y"=-32.00685516683127}, {"X"=632000.0, "Y"=-32.03435160349226}, {"X"=633000.0, "Y"=-32.061804662699885}, {"X"=634000.0, "Y"=-32.08921448049816}, {"X"=635000.0, "Y"=-32.11658119229332}, {"X"=636000.0, "Y"=-32.143904932859954}, {"X"=637000.0, "Y"=-32.171185836345316}, {"X"=638000.0, "Y"=-32.198424036273586}, {"X"=639000.0, "Y"=-32.22561966554755}, {"X"=640000.0, "Y"=-32.25277285645372}, {"X"=641000.0, "Y"=-32.27988374066634}, {"X"=642000.0, "Y"=-32.30695244925195}, {"X"=643000.0, "Y"=-32.33397911266803}, {"X"=644000.0, "Y"=-32.36096386077684}, {"X"=645000.0, "Y"=-32.38790682283795}, {"X"=646000.0, "Y"=-32.41480812751788}, {"X"=647000.0, "Y"=-32.441667902893656}, {"X"=648000.0, "Y"=-32.468486276454826}, {"X"=649000.0, "Y"=-32.495263375107484}, {"X"=650000.0, "Y"=-32.521999325179934}, {"X"=651000.0, "Y"=-32.548694252421186}, {"X"=652000.0, "Y"=-32.57534828200792}, {"X"=653000.0, "Y"=-32.60196153854959}, {"X"=654000.0, "Y"=-32.628534146087325}, {"X"=655000.0, "Y"=-32.655066228101035}, {"X"=656000.0, "Y"=-32.681557907511866}, {"X"=657000.0, "Y"=-32.70800930668423}, {"X"=658000.0, "Y"=-32.7344205474308}, {"X"=659000.0, "Y"=-32.760791751013286}, {"X"=660000.0, "Y"=-32.78712303814894}, {"X"=661000.0, "Y"=-32.81341452901403}, {"X"=662000.0, "Y"=-32.83966634324256}, {"X"=663000.0, "Y"=-32.86587859993502}, {"X"=664000.0, "Y"=-32.89205141765564}, {"X"=665000.0, "Y"=-32.918184914441014}, {"X"=666000.0, "Y"=-32.944279207802}, {"X"=667000.0, "Y"=-32.970334414723006}, {"X"=668000.0, "Y"=-32.99635065167007}, {"X"=669000.0, "Y"=-33.022328034592206}, {"X"=670000.0, "Y"=-33.04826667892203}, {"X"=671000.0, "Y"=-33.07416669958218}, {"X"=672000.0, "Y"=-33.10002821098654}, {"X"=673000.0, "Y"=-33.12585132704434}, {"X"=674000.0, "Y"=-33.151636161162386}, {"X"=675000.0, "Y"=-33.17738282624673}, {"X"=676000.0, "Y"=-33.20309143470692}, {"X"=677000.0, "Y"=-33.2287620984619}, {"X"=678000.0, "Y"=-33.25439492893559}, {"X"=679000.0, "Y"=-33.27999003706799}, {"X"=680000.0, "Y"=-33.305547533309706}, {"X"=681000.0, "Y"=-33.331067527633465}, {"X"=682000.0, "Y"=-33.35655012953054}, {"X"=683000.0, "Y"=-33.381995448015324}, {"X"=684000.0, "Y"=-33.40740359162794}, {"X"=685000.0, "Y"=-33.43277466843808}, {"X"=686000.0, "Y"=-33.45810878604801}, {"X"=687000.0, "Y"=-33.4834060515919}, {"X"=688000.0, "Y"=-33.50866657174157}, {"X"=689000.0, "Y"=-33.53389045270975}, {"X"=690000.0, "Y"=-33.559077800251444}, {"X"=691000.0, "Y"=-33.5842287196629}, {"X"=692000.0, "Y"=-33.60934331579291}, {"X"=693000.0, "Y"=-33.63442169303601}, {"X"=694000.0, "Y"=-33.659463955342396}, {"X"=695000.0, "Y"=-33.68447020621501}, {"X"=696000.0, "Y"=-33.70944054871575}, {"X"=697000.0, "Y"=-33.73437508546617}, {"X"=698000.0, "Y"=-33.75927391865054}, {"X"=699000.0, "Y"=-33.784137150021046}, {"X"=700000.0, "Y"=-33.80896488089067}, {"X"=701000.0, "Y"=-33.83375721214942}, {"X"=702000.0, "Y"=-33.85851424425688}, {"X"=703000.0, "Y"=-33.883236077246494}, {"X"=704000.0, "Y"=-33.90792281073152}, {"X"=705000.0, "Y"=-33.93257454390356}, {"X"=706000.0, "Y"=-33.95719137553364}, {"X"=707000.0, "Y"=-33.981773403982835}, {"X"=708000.0, "Y"=-34.00632072719253}, {"X"=709000.0, "Y"=-34.0308334426986}, {"X"=710000.0, "Y"=-34.05531164762503}, {"X"=711000.0, "Y"=-34.079755438690185}, {"X"=712000.0, "Y"=-34.10416491220821}, {"X"=713000.0, "Y"=-34.1285401640912}, {"X"=714000.0, "Y"=-34.15288128985085}, {"X"=715000.0, "Y"=-34.177188384604456}, {"X"=716000.0, "Y"=-34.20146154306826}, {"X"=717000.0, "Y"=-34.225700859572044}, {"X"=718000.0, "Y"=-34.249906428049314}, {"X"=719000.0, "Y"=-34.27407834204849}, {"X"=720000.0, "Y"=-34.29821669472832}, {"X"=721000.0, "Y"=-34.32232157886466}, {"X"=722000.0, "Y"=-34.346393086851904}, {"X"=723000.0, "Y"=-34.37043131070197}, {"X"=724000.0, "Y"=-34.39443634205136}, {"X"=725000.0, "Y"=-34.41840827215565}, {"X"=726000.0, "Y"=-34.44234719190124}, {"X"=727000.0, "Y"=-34.46625319180021}, {"X"=728000.0, "Y"=-34.49012636199532}, {"X"=729000.0, "Y"=-34.513966792259716}, {"X"=730000.0, "Y"=-34.5377745720032}, {"X"=731000.0, "Y"=-34.56154979026916}, {"X"=732000.0, "Y"=-34.585292535740976}, {"X"=733000.0, "Y"=-34.60900289673901}, {"X"=734000.0, "Y"=-34.63268096122832}, {"X"=735000.0, "Y"=-34.6563268168165}, {"X"=736000.0, "Y"=-34.67994055075644}, {"X"=737000.0, "Y"=-34.703522249949586}, {"X"=738000.0, "Y"=-34.72707200094726}, {"X"=739000.0, "Y"=-34.750589889950376}, {"X"=740000.0, "Y"=-34.77407600281428}, {"X"=741000.0, "Y"=-34.79753042504927}, {"X"=742000.0, "Y"=-34.82095324182218}, {"X"=743000.0, "Y"=-34.84434453796004}, {"X"=744000.0, "Y"=-34.86770439794934}, {"X"=745000.0, "Y"=-34.891032905937315}, {"X"=746000.0, "Y"=-34.91433014573913}, {"X"=747000.0, "Y"=-34.937596200833426}, {"X"=748000.0, "Y"=-34.960831154366836}, {"X"=749000.0, "Y"=-34.984035089155896}, {"X"=750000.0, "Y"=-35.00720808768863}, {"X"=751000.0, "Y"=-35.03035023212598}, {"X"=752000.0, "Y"=-35.05346160430253}, {"X"=753000.0, "Y"=-35.07654228573135}, {"X"=754000.0, "Y"=-35.09959235760228}, {"X"=755000.0, "Y"=-35.122611900784634}, {"X"=756000.0, "Y"=-35.14560099583096}, {"X"=757000.0, "Y"=-35.168559722974436}, {"X"=758000.0, "Y"=-35.19148816213515}, {"X"=759000.0, "Y"=-35.214386392920424}, {"X"=760000.0, "Y"=-35.23725449462225}, {"X"=761000.0, "Y"=-35.260092546226495}, {"X"=762000.0, "Y"=-35.28290062640817}, {"X"=763000.0, "Y"=-35.305678813533916}, {"X"=764000.0, "Y"=-35.32842718566891}, {"X"=765000.0, "Y"=-35.35114582057004}, {"X"=766000.0, "Y"=-35.37383479569569}, {"X"=767000.0, "Y"=-35.39649418820241}, {"X"=768000.0, "Y"=-35.419124074945216}, {"X"=769000.0, "Y"=-35.4417245324852}, {"X"=770000.0, "Y"=-35.46429563708464}, {"X"=771000.0, "Y"=-35.48683746471284}, {"X"=772000.0, "Y"=-35.50935009104589}, {"X"=773000.0, "Y"=-35.531833591467205}, {"X"=774000.0, "Y"=-35.554288041072446}, {"X"=775000.0, "Y"=-35.57671351466627}, {"X"=776000.0, "Y"=-35.59911008676665}, {"X"=777000.0, "Y"=-35.62147783160818}, {"X"=778000.0, "Y"=-35.64381682314034}, {"X"=779000.0, "Y"=-35.66612713502673}, {"X"=780000.0, "Y"=-35.68840884065494}, {"X"=781000.0, "Y"=-35.71066201312893}, {"X"=782000.0, "Y"=-35.73288672527632}, {"X"=783000.0, "Y"=-35.75508304964706}, {"X"=784000.0, "Y"=-35.77725105851456}, {"X"=785000.0, "Y"=-35.799390823879}, {"X"=786000.0, "Y"=-35.82150241746765}, {"X"=787000.0, "Y"=-35.843585910737666}, {"X"=788000.0, "Y"=-35.86564137487443}, {"X"=789000.0, "Y"=-35.8876688807939}, {"X"=790000.0, "Y"=-35.90966849914688}, {"X"=791000.0, "Y"=-35.931640300317156}, {"X"=792000.0, "Y"=-35.953584354423135}, {"X"=793000.0, "Y"=-35.975500731322256}, {"X"=794000.0, "Y"=-35.99738950060656}, {"X"=795000.0, "Y"=-36.01925073160953}, {"X"=796000.0, "Y"=-36.04108449340625}, {"X"=797000.0, "Y"=-36.0628908548095}, {"X"=798000.0, "Y"=-36.084669884381455}, {"X"=799000.0, "Y"=-36.106421650422}, {"X"=800000.0, "Y"=-36.128146220981456}, {"X"=801000.0, "Y"=-36.14984366385662}, {"X"=802000.0, "Y"=-36.17151404658949}, {"X"=803000.0, "Y"=-36.19315743647521}, {"X"=804000.0, "Y"=-36.21477390055571}, {"X"=805000.0, "Y"=-36.236363505630194}, {"X"=806000.0, "Y"=-36.257926318246916}, {"X"=807000.0, "Y"=-36.27946240470874}, {"X"=808000.0, "Y"=-36.300971831074506}, {"X"=809000.0, "Y"=-36.322454663161494}, {"X"=810000.0, "Y"=-36.34391096654321}, {"X"=811000.0, "Y"=-36.36534080655228}, {"X"=812000.0, "Y"=-36.386744248283044}, {"X"=813000.0, "Y"=-36.408121356591494}, {"X"=814000.0, "Y"=-36.42947219609195}, {"X"=815000.0, "Y"=-36.450796831168816}, {"X"=816000.0, "Y"=-36.47209532596777}, {"X"=817000.0, "Y"=-36.49336774440117}, {"X"=818000.0, "Y"=-36.514614150148944}, {"X"=819000.0, "Y"=-36.53583460665833}, {"X"=820000.0, "Y"=-36.557029177148024}, {"X"=821000.0, "Y"=-36.578197924606975}, {"X"=822000.0, "Y"=-36.599340911793874}, {"X"=823000.0, "Y"=-36.62045820124259}, {"X"=824000.0, "Y"=-36.641549855259036}, {"X"=825000.0, "Y"=-36.66261593592504}, {"X"=826000.0, "Y"=-36.683656505098526}, {"X"=827000.0, "Y"=-36.704671624415504}, {"X"=828000.0, "Y"=-36.725661355288615}, {"X"=829000.0, "Y"=-36.74662575890985}, {"X"=830000.0, "Y"=-36.76756489625183}, {"X"=831000.0, "Y"=-36.78847882807084}, {"X"=832000.0, "Y"=-36.80936761490137}, {"X"=833000.0, "Y"=-36.83023131706547}, {"X"=834000.0, "Y"=-36.85106999466678}, {"X"=835000.0, "Y"=-36.87188370759526}, {"X"=836000.0, "Y"=-36.89267251552786}, {"X"=837000.0, "Y"=-36.91343647792946}, {"X"=838000.0, "Y"=-36.93417565405276}, {"X"=839000.0, "Y"=-36.954890102940226}, {"X"=840000.0, "Y"=-36.975579883426036}, {"X"=841000.0, "Y"=-36.99624505413273}, {"X"=842000.0, "Y"=-37.01688567347979}, {"X"=843000.0, "Y"=-37.03750179967538}, {"X"=844000.0, "Y"=-37.05809349072703}, {"X"=845000.0, "Y"=-37.07866080443273}, {"X"=846000.0, "Y"=-37.09920379839141}, {"X"=847000.0, "Y"=-37.119722529997176}, {"X"=848000.0, "Y"=-37.14021705644301}, {"X"=849000.0, "Y"=-37.16068743472072}, {"X"=850000.0, "Y"=-37.181133721621926}, {"X"=851000.0, "Y"=-37.20155597373949}, {"X"=852000.0, "Y"=-37.22195424746935}, {"X"=853000.0, "Y"=-37.24232859901034}, {"X"=854000.0, "Y"=-37.26267908436405}, {"X"=855000.0, "Y"=-37.2830057593375}, {"X"=856000.0, "Y"=-37.30330867954223}, {"X"=857000.0, "Y"=-37.32358790039974}, {"X"=858000.0, "Y"=-37.343843477136105}, {"X"=859000.0, "Y"=-37.36407546478449}, {"X"=860000.0, "Y"=-37.38428391819129}, {"X"=861000.0, "Y"=-37.40446889201114}, {"X"=862000.0, "Y"=-37.42463044070937}, {"X"=863000.0, "Y"=-37.44476861856271}, {"X"=864000.0, "Y"=-37.46488347966201}, {"X"=865000.0, "Y"=-37.484975077910676}, {"X"=866000.0, "Y"=-37.50504346702802}, {"X"=867000.0, "Y"=-37.52508870054576}, {"X"=868000.0, "Y"=-37.54511083181569}, {"X"=869000.0, "Y"=-37.565109914003074}, {"X"=870000.0, "Y"=-37.585086000094186}, {"X"=871000.0, "Y"=-37.605039142891016}, {"X"=872000.0, "Y"=-37.62496939501724}, {"X"=873000.0, "Y"=-37.64487680891438}, {"X"=874000.0, "Y"=-37.66476143684814}, {"X"=875000.0, "Y"=-37.68462333090458}, {"X"=876000.0, "Y"=-37.70446254299268}, {"X"=877000.0, "Y"=-37.724279124842866}, {"X"=878000.0, "Y"=-37.74407312801464}, {"X"=879000.0, "Y"=-37.76384460388844}, {"X"=880000.0, "Y"=-37.78359360367241}, {"X"=881000.0, "Y"=-37.803320178401464}, {"X"=882000.0, "Y"=-37.82302437893674}, {"X"=883000.0, "Y"=-37.84270625596874}, {"X"=884000.0, "Y"=-37.86236586001809}, {"X"=885000.0, "Y"=-37.882003241431946}, {"X"=886000.0, "Y"=-37.90161845039118}, {"X"=887000.0, "Y"=-37.921211536907016}, {"X"=888000.0, "Y"=-37.94078255082201}, {"X"=889000.0, "Y"=-37.96033154181262}, {"X"=890000.0, "Y"=-37.979858559387225}, {"X"=891000.0, "Y"=-37.99936365289001}, {"X"=892000.0, "Y"=-38.01884687149937}, {"X"=893000.0, "Y"=-38.03830826423149}, {"X"=894000.0, "Y"=-38.05774787993641}, {"X"=895000.0, "Y"=-38.07716576730114}, {"X"=896000.0, "Y"=-38.096561974854524}, {"X"=897000.0, "Y"=-38.115936550959205}, {"X"=898000.0, "Y"=-38.1352895438213}, {"X"=899000.0, "Y"=-38.15462100148315}, {"X"=900000.0, "Y"=-38.17393097183154}, {"X"=901000.0, "Y"=-38.19321950259302}, {"X"=902000.0, "Y"=-38.21248664133665}, {"X"=903000.0, "Y"=-38.23173243547173}, {"X"=904000.0, "Y"=-38.25095693225712}, {"X"=905000.0, "Y"=-38.27016017879027}, {"X"=906000.0, "Y"=-38.28934222201606}, {"X"=907000.0, "Y"=-38.30850310872404}, {"X"=908000.0, "Y"=-38.32764288555089}, {"X"=909000.0, "Y"=-38.34676159898148}, {"X"=910000.0, "Y"=-38.365859295344535}, {"X"=911000.0, "Y"=-38.384936020820845}, {"X"=912000.0, "Y"=-38.40399182143757}, {"X"=913000.0, "Y"=-38.42302674307404}, {"X"=914000.0, "Y"=-38.442040831456744}, {"X"=915000.0, "Y"=-38.46103413216501}, {"X"=916000.0, "Y"=-38.48000669062902}, {"X"=917000.0, "Y"=-38.498958552133764}, {"X"=918000.0, "Y"=-38.51788976181234}, {"X"=919000.0, "Y"=-38.53680036465449}, {"X"=920000.0, "Y"=-38.55569040550348}, {"X"=921000.0, "Y"=-38.57455992905718}, {"X"=922000.0, "Y"=-38.59340897986806}, {"X"=923000.0, "Y"=-38.612237602346255}, {"X"=924000.0, "Y"=-38.63104584075735}, {"X"=925000.0, "Y"=-38.64983373922364}, {"X"=926000.0, "Y"=-38.66860134172683}, {"X"=927000.0, "Y"=-38.68734869210455}, {"X"=928000.0, "Y"=-38.70607583405688}, {"X"=929000.0, "Y"=-38.72478281114147}, {"X"=930000.0, "Y"=-38.743469666774544}, {"X"=931000.0, "Y"=-38.762136444237015}, {"X"=932000.0, "Y"=-38.78078318666863}, {"X"=933000.0, "Y"=-38.799409937070884}, {"X"=934000.0, "Y"=-38.81801673830884}, {"X"=935000.0, "Y"=-38.836603633112276}, {"X"=936000.0, "Y"=-38.8551706640712}, {"X"=937000.0, "Y"=-38.87371787364255}, {"X"=938000.0, "Y"=-38.89224530414631}, {"X"=939000.0, "Y"=-38.910752997769926}, {"X"=940000.0, "Y"=-38.92924099656584}, {"X"=941000.0, "Y"=-38.947709342453216}, {"X"=942000.0, "Y"=-38.9661580772181}, {"X"=943000.0, "Y"=-38.98458724251506}, {"X"=944000.0, "Y"=-39.002996879865506}, {"X"=945000.0, "Y"=-39.021387030661245}, {"X"=946000.0, "Y"=-39.039757736162656}, {"X"=947000.0, "Y"=-39.058109037500614}, {"X"=948000.0, "Y"=-39.0764409756757}, {"X"=949000.0, "Y"=-39.094753591559474}, {"X"=950000.0, "Y"=-39.113046925895034}, {"X"=951000.0, "Y"=-39.131321019298696}, {"X"=952000.0, "Y"=-39.149575912257895}, {"X"=953000.0, "Y"=-39.16781164513569}, {"X"=954000.0, "Y"=-39.186028258163844}, {"X"=955000.0, "Y"=-39.20422579145437}, {"X"=956000.0, "Y"=-39.22240428499097}, {"X"=957000.0, "Y"=-39.2405637786313}, {"X"=958000.0, "Y"=-39.25870431211121}, {"X"=959000.0, "Y"=-39.27682592504113}, {"X"=960000.0, "Y"=-39.294928656909256}, {"X"=961000.0, "Y"=-39.31301254708198}, {"X"=962000.0, "Y"=-39.3310776348001}, {"X"=963000.0, "Y"=-39.34912395918588}, {"X"=964000.0, "Y"=-39.36715155924}, {"X"=965000.0, "Y"=-39.38516047384183}, {"X"=966000.0, "Y"=-39.40315074174873}, {"X"=967000.0, "Y"=-39.421122401601075}, {"X"=968000.0, "Y"=-39.43907549191873}, {"X"=969000.0, "Y"=-39.45701005110523}, {"X"=970000.0, "Y"=-39.47492611744145}, {"X"=971000.0, "Y"=-39.4928237290938}, {"X"=972000.0, "Y"=-39.51070292410969}, {"X"=973000.0, "Y"=-39.528563740420395}, {"X"=974000.0, "Y"=-39.5464062158421}, {"X"=975000.0, "Y"=-39.564230388071884}, {"X"=976000.0, "Y"=-39.582036294695015}, {"X"=977000.0, "Y"=-39.59982397318008}, {"X"=978000.0, "Y"=-39.61759346087939}, {"X"=979000.0, "Y"=-39.635344795036424}, {"X"=980000.0, "Y"=-39.65307801277446}, {"X"=981000.0, "Y"=-39.670793151109585}, {"X"=982000.0, "Y"=-39.68849024694282}, {"X"=983000.0, "Y"=-39.70616933706126}, {"X"=984000.0, "Y"=-39.72383045814176}, {"X"=985000.0, "Y"=-39.74147364675355}, {"X"=986000.0, "Y"=-39.75909893934698}, {"X"=987000.0, "Y"=-39.776706372269935}, {"X"=988000.0, "Y"=-39.79429598175621}, {"X"=989000.0, "Y"=-39.81186780393026}, {"X"=990000.0, "Y"=-39.82942187480929}, {"X"=991000.0, "Y"=-39.84695823029936}, {"X"=992000.0, "Y"=-39.8644769062003}, {"X"=993000.0, "Y"=-39.88197793820579}, {"X"=994000.0, "Y"=-39.899461361896876}, {"X"=995000.0, "Y"=-39.91692721275173}, {"X"=996000.0, "Y"=-39.93437552614163}, {"X"=997000.0, "Y"=-39.95180633733152}, {"X"=998000.0, "Y"=-39.96921968148011}, {"X"=999000.0, "Y"=-39.98661559364272}, {"X"=1000000.0, "Y"=-40.00399410876531}]
  out "Phase":cluster{"X":dbl, "Y":dbl}[](graph)=[{"X"=1000.0, "Y"=-5.684341886080802e-14}, {"X"=2000.0, "Y"=-5.684341886080802e-14}, {"X"=3000.0, "Y"=-1.470338854782966}, {"X"=4000.0, "Y"=-2.5472600369326983}, {"X"=5000.0, "Y"=-3.507032968301246}, {"X"=6000.0, "Y"=-4.41488111814121}, {"X"=7000.0, "Y"=-5.295187660987267}, {"X"=8000.0, "Y"=-6.159363304359161}, {"X"=9000.0, "Y"=-7.013548001936471}, {"X"=10000.0, "Y"=-7.861386359435812}, {"X"=11000.0, "Y"=-8.705209477045031}, {"X"=12000.0, "Y"=-9.546600438357359}, {"X"=13000.0, "Y"=-10.38668940710977}, {"X"=14000.0, "Y"=-11.22631835206522}, {"X"=15000.0, "Y"=-12.066138090435615}, {"X"=16000.0, "Y"=-12.906668035974548}, {"X"=17000.0, "Y"=-13.748334357682722}, {"X"=18000.0, "Y"=-14.591495111348152}, {"X"=19000.0, "Y"=-15.436457226322446}, {"X"=20000.0, "Y"=-16.283488240889966}, {"X"=21000.0, "Y"=-17.13282455910931}, {"X"=22000.0, "Y"=-17.984677347693378}, {"X"=23000.0, "Y"=-18.839236797204194}, {"X"=24000.0, "Y"=-19.696675227495263}, {"X"=25000.0, "Y"=-20.55714936212027}, {"X"=26000.0, "Y"=-21.42080199560067}, {"X"=27000.0, "Y"=-22.287763210635887}, {"X"=28000.0, "Y"=-23.158151257253593}, {"X"=29000.0, "Y"=-24.032073174981008}, {"X"=30000.0, "Y"=-24.909625217597068}, {"X"=31000.0, "Y"=-25.790893124867182}, {"X"=32000.0, "Y"=-26.67595227481638}, {"X"=33000.0, "Y"=-27.56486774233629}, {"X"=34000.0, "Y"=-28.457694284219528}, {"X"=35000.0, "Y"=-29.35447626661184}, {"X"=36000.0, "Y"=-30.255247547801133}, {"X"=37000.0, "Y"=-31.160031327042105}, {"X"=38000.0, "Y"=-32.06883996845926}, {"X"=39000.0, "Y"=-32.981674807848535}, {"X"=40000.0, "Y"=-33.89852594933416}, {"X"=41000.0, "Y"=-34.819372058163424}, {"X"=42000.0, "Y"=-35.744180155477125}, {"X"=43000.0, "Y"=-36.67290542054319}, {"X"=44000.0, "Y"=-37.6054910056952}, {"X"=45000.0, "Y"=-38.541867869036935}, {"X"=46000.0, "Y"=-39.48195462980769}, {"X"=47000.0, "Y"=-40.425657451168405}, {"X"=48000.0, "Y"=-41.37286995500821}, {"X"=49000.0, "Y"=-42.32347317321276}, {"X"=50000.0, "Y"=-43.277335539619884}, {"X"=51000.0, "Y"=-44.234312926597994}, {"X"=52000.0, "Y"=-45.1942487299502}, {"X"=53000.0, "Y"=-46.15697400538005}, {"X"=54000.0, "Y"=-47.09453809673346}, {"X"=55000.0, "Y"=-48.06059722718146}, {"X"=56000.0, "Y"=-49.02889012037127}, {"X"=57000.0, "Y"=-49.99921922628707}, {"X"=58000.0, "Y"=-50.97137778044515}, {"X"=59000.0, "Y"=-51.94515022141408}, {"X"=60000.0, "Y"=-52.9203126431305}, {"X"=61000.0, "Y"=-53.896633280215525}, {"X"=62000.0, "Y"=-54.87387302423949}, {"X"=63000.0, "Y"=-55.85178596860794}, {"X"=64000.0, "Y"=-56.83011997944854}, {"X"=65000.0, "Y"=-57.8086172897257}, {"X"=66000.0, "Y"=-58.78701511359358}, {"X"=67000.0, "Y"=-59.76504627782123}, {"X"=68000.0, "Y"=-60.74243986711036}, {"X"=69000.0, "Y"=-61.71892187993171}, {"X"=70000.0, "Y"=-62.694215891576704}, {"X"=71000.0, "Y"=-63.6680437210436}, {"X"=72000.0, "Y"=-64.6401260984529}, {"X"=73000.0, "Y"=-65.61018332975925}, {"X"=74000.0, "Y"=-66.57793595556399}, {"X"=75000.0, "Y"=-67.54310540102384}, {"X"=76000.0, "Y"=-68.50541461394874}, {"X"=77000.0, "Y"=-69.46458868839326}, {"X"=78000.0, "Y"=-70.42035547109302}, {"X"=79000.0, "Y"=-71.37244614854825}, {"X"=80000.0, "Y"=-72.32059581240526}, {"X"=81000.0, "Y"=-73.26454400136504}, {"X"=82000.0, "Y"=-74.20403521773679}, {"X"=83000.0, "Y"=-75.13881941719376}, {"X"=84000.0, "Y"=-76.0686524703928}, {"X"=85000.0, "Y"=-76.99329659528806}, {"X"=86000.0, "Y"=-77.91252075935412}, {"X"=87000.0, "Y"=-78.82610105084677}, {"X"=88000.0, "Y"=-79.73382101873813}, {"X"=89000.0, "Y"=-80.6354719808229}, {"X"=90000.0, "Y"=-81.53085329998723}, {"X"=91000.0, "Y"=-82.41977262845634}, {"X"=92000.0, "Y"=-83.30204612035175}, {"X"=93000.0, "Y"=-84.17749861267629}, {"X"=94000.0, "Y"=-84.96831391947836}, {"X"=95000.0, "Y"=-85.82678505988164}, {"X"=96000.0, "Y"=-86.67801326451351}, {"X"=97000.0, "Y"=-87.521868017061}, {"X"=98000.0, "Y"=-88.35822768984016}, {"X"=99000.0, "Y"=-89.18697950427094}, {"X"=100000.0, "Y"=-90.00801946878852}, {"X"=101000.0, "Y"=-90.82125229545}, {"X"=102000.0, "Y"=-91.62659129675683}, {"X"=103000.0, "Y"=-92.42395826391544}, {"X"=104000.0, "Y"=-93.21328332807445}, {"X"=105000.0, "Y"=-93.99450480578594}, {"X"=106000.0, "Y"=-94.76756903010397}, {"X"=107000.0, "Y"=-95.53243016857903}, {"X"=108000.0, "Y"=-96.28905002947766}, {"X"=109000.0, "Y"=-97.03739785751043}, {"X"=110000.0, "Y"=-97.77745012022172}, {"X"=111000.0, "Y"=-98.5091902862967}, {"X"=112000.0, "Y"=-99.23260859686843}, {"X"=113000.0, "Y"=-99.9477018310543}, {"X"=114000.0, "Y"=-100.65447306660843}, {"X"=115000.0, "Y"=-101.3529314368925}, {"X"=116000.0, "Y"=-102.04309188499218}, {"X"=117000.0, "Y"=-102.72497491602888}, {"X"=118000.0, "Y"=-103.3986063484615}, {"X"=119000.0, "Y"=-104.06401706523533}, {"X"=120000.0, "Y"=-104.72124276560814}, {"X"=121000.0, "Y"=-105.37032371831526}, {"X"=122000.0, "Y"=-106.01130451677929}, {"X"=123000.0, "Y"=-106.30151609358569}, {"X"=124000.0, "Y"=-106.91261232944586}, {"X"=125000.0, "Y"=-107.51585930386096}, {"X"=126000.0, "Y"=-108.1113309562704}, {"X"=127000.0, "Y"=-108.69910360164982}, {"X"=128000.0, "Y"=-109.27925570470185}, {"X"=129000.0, "Y"=-109.85186766347414}, {"X"=130000.0, "Y"=-110.41702160226183}, {"X"=131000.0, "Y"=-110.9748011739126}, {"X"=132000.0, "Y"=-111.52529137145262}, {"X"=133000.0, "Y"=-112.0685783488396}, {"X"=134000.0, "Y"=-112.60474925085302}, {"X"=135000.0, "Y"=-113.13389205187195}, {"X"=136000.0, "Y"=-113.65609540340111}, {"X"=137000.0, "Y"=-114.17144849015259}, {"X"=138000.0, "Y"=-114.68004089441544}, {"X"=139000.0, "Y"=-115.18196246855297}, {"X"=140000.0, "Y"=-115.67730321533813}, {"X"=141000.0, "Y"=-116.16615317587403}, {"X"=142000.0, "Y"=-116.64860232481891}, {"X"=143000.0, "Y"=-117.12474047270032}, {"X"=144000.0, "Y"=-117.59465717500811}, {"X"=145000.0, "Y"=-118.05844164778989}, {"X"=146000.0, "Y"=-118.51618268945757}, {"X"=147000.0, "Y"=-118.96796860860417}, {"X"=148000.0, "Y"=-119.41388715744998}, {"X"=149000.0, "Y"=-119.85402547074213}, {"X"=150000.0, "Y"=-120.28847000979067}, {"X"=151000.0, "Y"=-120.71730651142647}, {"X"=152000.0, "Y"=-121.14061994151115}, {"X"=153000.0, "Y"=-121.55849445294314}, {"X"=154000.0, "Y"=-121.97101334776019}, {"X"=155000.0, "Y"=-122.37825904313999}, {"X"=156000.0, "Y"=-122.78031304110917}, {"X"=157000.0, "Y"=-123.17725590175831}, {"X"=158000.0, "Y"=-123.56916721963375}, {"X"=159000.0, "Y"=-123.95612560328374}, {"X"=160000.0, "Y"=-124.33820865760939}, {"X"=161000.0, "Y"=-124.71549296889688}, {"X"=162000.0, "Y"=-125.08805409239477}, {"X"=163000.0, "Y"=-125.45596654218181}, {"X"=164000.0, "Y"=-125.81930378324057}, {"X"=165000.0, "Y"=-126.17813822551011}, {"X"=166000.0, "Y"=-126.53254121987982}, {"X"=167000.0, "Y"=-126.88258305584606}, {"X"=168000.0, "Y"=-127.22833296081657}, {"X"=169000.0, "Y"=-127.56985910091385}, {"X"=170000.0, "Y"=-127.90722858307348}, {"X"=171000.0, "Y"=-128.2405074584957}, {"X"=172000.0, "Y"=-128.56976072714792}, {"X"=173000.0, "Y"=-128.89505234341385}, {"X"=174000.0, "Y"=-129.21644522261002}, {"X"=175000.0, "Y"=-129.53400124846763}, {"X"=176000.0, "Y"=-129.84778128135179}, {"X"=177000.0, "Y"=-130.1578451671919}, {"X"=178000.0, "Y"=-130.46425174710674}, {"X"=179000.0, "Y"=-130.7670588675739}, {"X"=180000.0, "Y"=-131.06632339111127}, {"X"=181000.0, "Y"=-131.36210120745528}, {"X"=182000.0, "Y"=-131.65444724508953}, {"X"=183000.0, "Y"=-131.94341548319096}, {"X"=184000.0, "Y"=-132.22905896381707}, {"X"=185000.0, "Y"=-132.5114298044458}, {"X"=186000.0, "Y"=-132.79057921062258}, {"X"=187000.0, "Y"=-133.06655748892456}, {"X"=188000.0, "Y"=-133.3394140599608}, {"X"=189000.0, "Y"=-133.6091974715657}, {"X"=190000.0, "Y"=-133.87595541207997}, {"X"=191000.0, "Y"=-134.13973472363435}, {"X"=192000.0, "Y"=-134.4005814155535}, {"X"=193000.0, "Y"=-134.65854067772995}, {"X"=194000.0, "Y"=-134.91365689397406}, {"X"=195000.0, "Y"=-135.16597365540594}, {"X"=196000.0, "Y"=-135.41553377372105}, {"X"=197000.0, "Y"=-135.6623792944846}, {"X"=198000.0, "Y"=-135.90655151026613}, {"X"=199000.0, "Y"=-136.14809097375723}, {"X"=200000.0, "Y"=-136.38703751076193}, {"X"=201000.0, "Y"=-136.62343023306934}, {"X"=202000.0, "Y"=-136.85730755121386}, {"X"=203000.0, "Y"=-137.08870718713484}, {"X"=204000.0, "Y"=-137.3176661866636}, {"X"=205000.0, "Y"=-137.54422093186113}, {"X"=206000.0, "Y"=-137.76840715327015}, {"X"=207000.0, "Y"=-137.99025994193826}, {"X"=208000.0, "Y"=-138.2098137613319}, {"X"=209000.0, "Y"=-138.42710245905835}, {"X"=210000.0, "Y"=-138.64215927846112}, {"X"=211000.0, "Y"=-138.85501686999032}, {"X"=212000.0, "Y"=-139.06570730245164}, {"X"=213000.0, "Y"=-139.27426207406833}, {"X"=214000.0, "Y"=-139.4807121233421}, {"X"=215000.0, "Y"=-139.68508783979178}, {"X"=216000.0, "Y"=-139.88741907446337}, {"X"=217000.0, "Y"=-140.0877351502902}, {"X"=218000.0, "Y"=-140.2860648722893}, {"X"=219000.0, "Y"=-140.48243653753806}, {"X"=220000.0, "Y"=-140.67687794503178}, {"X"=221000.0, "Y"=-140.86941640532356}, {"X"=222000.0, "Y"=-141.06007875000427}, {"X"=223000.0, "Y"=-141.24889134102014}, {"X"=224000.0, "Y"=-141.43588007979432}, {"X"=225000.0, "Y"=-141.62107041622204}, {"X"=226000.0, "Y"=-141.80448735742604}, {"X"=227000.0, "Y"=-141.9861554764334}, {"X"=228000.0, "Y"=-142.1660989206149}, {"X"=229000.0, "Y"=-142.34434142001712}, {"X"=230000.0, "Y"=-142.52090629546962}, {"X"=231000.0, "Y"=-142.6958164666039}, {"X"=232000.0, "Y"=-142.86909445966035}, {"X"=233000.0, "Y"=-143.0407624151851}, {"X"=234000.0, "Y"=-143.21084209554016}, {"X"=235000.0, "Y"=-143.37935489227655}, {"X"=236000.0, "Y"=-143.54632183335843}, {"X"=237000.0, "Y"=-143.71176359025586}, {"X"=238000.0, "Y"=-143.87570048486856}, {"X"=239000.0, "Y"=-144.0381524963393}, {"X"=240000.0, "Y"=-144.19913926770346}, {"X"=241000.0, "Y"=-144.35868011241436}, {"X"=242000.0, "Y"=-144.51679402073833}, {"X"=243000.0, "Y"=-144.67349966601466}, {"X"=244000.0, "Y"=-144.82881541078433}, {"X"=245000.0, "Y"=-144.98275931280872}, {"X"=246000.0, "Y"=-145.13534913093036}, {"X"=247000.0, "Y"=-145.2866023308616}, {"X"=248000.0, "Y"=-145.4365360908044}, {"X"=249000.0, "Y"=-145.58516730698236}, {"X"=250000.0, "Y"=-145.73251259906274}, {"X"=251000.0, "Y"=-145.8785883154493}, {"X"=252000.0, "Y"=-146.02341053845652}, {"X"=253000.0, "Y"=-146.16699508942003}, {"X"=254000.0, "Y"=-146.30935753365142}, {"X"=255000.0, "Y"=-146.45051318531023}, {"X"=256000.0, "Y"=-146.59047711219839}, {"X"=257000.0, "Y"=-146.72926414040177}, {"X"=258000.0, "Y"=-146.86688885888404}, {"X"=259000.0, "Y"=-147.00336562396507}, {"X"=260000.0, "Y"=-147.13870856369786}, {"X"=261000.0, "Y"=-147.27293158218035}, {"X"=262000.0, "Y"=-147.4060483637363}, {"X"=263000.0, "Y"=-147.53807237706388}, {"X"=264000.0, "Y"=-147.66901687924937}, {"X"=265000.0, "Y"=-147.79889491971574}, {"X"=266000.0, "Y"=-147.92771934410476}, {"X"=267000.0, "Y"=-148.05550279804518}, {"X"=268000.0, "Y"=-148.1822577308792}, {"X"=269000.0, "Y"=-148.30799639928247}, {"X"=270000.0, "Y"=-148.43273087082144}, {"X"=271000.0, "Y"=-148.55647302744103}, {"X"=272000.0, "Y"=-148.67923456887902}, {"X"=273000.0, "Y"=-148.8010270159953}, {"X"=274000.0, "Y"=-148.92186171405507}, {"X"=275000.0, "Y"=-149.04174983591997}, {"X"=276000.0, "Y"=-149.16070238521073}, {"X"=277000.0, "Y"=-149.27873019935413}, {"X"=278000.0, "Y"=-149.39584395260906}, {"X"=279000.0, "Y"=-149.51205415901273}, {"X"=280000.0, "Y"=-149.62737117526817}, {"X"=281000.0, "Y"=-149.74180520358365}, {"X"=282000.0, "Y"=-149.85536629443476}, {"X"=283000.0, "Y"=-149.96806434927723}, {"X"=284000.0, "Y"=-150.0799091232148}, {"X"=285000.0, "Y"=-150.1909102276108}, {"X"=286000.0, "Y"=-150.3010771326288}, {"X"=287000.0, "Y"=-150.41041916974794}, {"X"=288000.0, "Y"=-150.5189455341995}, {"X"=289000.0, "Y"=-150.6266652873874}, {"X"=290000.0, "Y"=-150.7335873592211}, {"X"=291000.0, "Y"=-150.83972055044015}, {"X"=292000.0, "Y"=-150.94507353486944}, {"X"=293000.0, "Y"=-151.04965486161953}, {"X"=294000.0, "Y"=-151.1534729572786}, {"X"=295000.0, "Y"=-151.256536128031}, {"X"=296000.0, "Y"=-151.35885256173188}, {"X"=297000.0, "Y"=-151.46043032996974}, {"X"=298000.0, "Y"=-151.56127739005632}, {"X"=299000.0, "Y"=-151.6614015869878}, {"X"=300000.0, "Y"=-151.76081065538145}, {"X"=301000.0, "Y"=-151.8595122213482}, {"X"=302000.0, "Y"=-151.95751380435456}, {"X"=303000.0, "Y"=-152.0548228190279}, {"X"=304000.0, "Y"=-152.15144657693043}, {"X"=305000.0, "Y"=-152.24739228831163}, {"X"=306000.0, "Y"=-152.34266706381302}, {"X"=307000.0, "Y"=-152.43727791613856}, {"X"=308000.0, "Y"=-152.53123176170044}, {"X"=309000.0, "Y"=-152.62453542223378}, {"X"=310000.0, "Y"=-152.71719562637782}, {"X"=311000.0, "Y"=-152.8092190112139}, {"X"=312000.0, "Y"=-152.90061212378842}, {"X"=313000.0, "Y"=-152.99138142261842}, {"X"=314000.0, "Y"=-153.08153327912845}, {"X"=315000.0, "Y"=-153.1710739791006}, {"X"=316000.0, "Y"=-153.26000972407843}, {"X"=317000.0, "Y"=-153.348346632742}, {"X"=318000.0, "Y"=-153.43609074226725}, {"X"=319000.0, "Y"=-153.52324800964317}, {"X"=320000.0, "Y"=-153.60982431298325}, {"X"=321000.0, "Y"=-153.69582545280224}, {"X"=322000.0, "Y"=-153.78125715326303}, {"X"=323000.0, "Y"=-153.86612506341993}, {"X"=324000.0, "Y"=-153.95043475841368}, {"X"=325000.0, "Y"=-154.0341917406495}, {"X"=326000.0, "Y"=-154.1174014409849}, {"X"=327000.0, "Y"=-154.20006921984526}, {"X"=328000.0, "Y"=-154.2822003683582}, {"X"=329000.0, "Y"=-154.36380010944384}, {"X"=330000.0, "Y"=-154.44487359889777}, {"X"=331000.0, "Y"=-154.52542592644375}, {"X"=332000.0, "Y"=-154.6054621167836}, {"X"=333000.0, "Y"=-154.68498713060927}, {"X"=334000.0, "Y"=-154.76400586560294}, {"X"=335000.0, "Y"=-154.8425231574206}, {"X"=336000.0, "Y"=-154.92054378066587}, {"X"=337000.0, "Y"=-154.99807244982497}, {"X"=338000.0, "Y"=-155.07511382020317}, {"X"=339000.0, "Y"=-155.1516724888416}, {"X"=340000.0, "Y"=-155.22775299540604}, {"X"=341000.0, "Y"=-155.3033598230788}, {"X"=342000.0, "Y"=-155.3784973993993}, {"X"=343000.0, "Y"=-155.45317009715384}, {"X"=344000.0, "Y"=-155.52738223517434}, {"X"=345000.0, "Y"=-155.6011380791713}, {"X"=346000.0, "Y"=-155.67444184254074}, {"X"=347000.0, "Y"=-155.7472976871511}, {"X"=348000.0, "Y"=-155.8197097241183}, {"X"=349000.0, "Y"=-155.89168201457193}, {"X"=350000.0, "Y"=-155.9632185704041}, {"X"=351000.0, "Y"=-156.03432335500736}, {"X"=352000.0, "Y"=-156.1050002839932}, {"X"=353000.0, "Y"=-156.17525322589773}, {"X"=354000.0, "Y"=-156.24508600289897}, {"X"=355000.0, "Y"=-156.31450239148407}, {"X"=356000.0, "Y"=-156.38350612312962}, {"X"=357000.0, "Y"=-156.45210088497475}, {"X"=358000.0, "Y"=-156.52029032044885}, {"X"=359000.0, "Y"=-156.58807802992825}, {"X"=360000.0, "Y"=-156.65546757136897}, {"X"=361000.0, "Y"=-156.72246246091015}, {"X"=362000.0, "Y"=-156.78906617348895}, {"X"=363000.0, "Y"=-156.85528214343762}, {"X"=364000.0, "Y"=-156.92111376506867}, {"X"=365000.0, "Y"=-156.986564393256}, {"X"=366000.0, "Y"=-157.0516373439953}, {"X"=367000.0, "Y"=-157.11633589496319}, {"X"=368000.0, "Y"=-157.18066328607426}, {"X"=369000.0, "Y"=-157.24462272000335}, {"X"=370000.0, "Y"=-157.30821736272884}, {"X"=371000.0, "Y"=-157.37145034405256}, {"X"=372000.0, "Y"=-157.4343247581012}, {"X"=373000.0, "Y"=-157.49684366384025}, {"X"=374000.0, "Y"=-157.55901008557106}, {"X"=375000.0, "Y"=-157.6208270134013}, {"X"=376000.0, "Y"=-157.68229740374937}, {"X"=377000.0, "Y"=-157.7434241797948}, {"X"=378000.0, "Y"=-157.80421023194452}, {"X"=379000.0, "Y"=-157.86465841829653}, {"X"=380000.0, "Y"=-157.92477156508693}, {"X"=381000.0, "Y"=-157.98455246712172}, {"X"=382000.0, "Y"=-158.04400388822114}, {"X"=383000.0, "Y"=-158.10312856163853}, {"X"=384000.0, "Y"=-158.1619291904783}, {"X"=385000.0, "Y"=-158.2204084481242}, {"X"=386000.0, "Y"=-158.2785689786266}, {"X"=387000.0, "Y"=-158.33641339710783}, {"X"=388000.0, "Y"=-158.3939442901656}, {"X"=389000.0, "Y"=-158.4511642162426}, {"X"=390000.0, "Y"=-158.50807570601916}, {"X"=391000.0, "Y"=-158.56468126279185}, {"X"=392000.0, "Y"=-158.62098336281815}, {"X"=393000.0, "Y"=-158.67698445571273}, {"X"=394000.0, "Y"=-158.7326869647768}, {"X"=395000.0, "Y"=-158.7880932873628}, {"X"=396000.0, "Y"=-158.8432057952136}, {"X"=397000.0, "Y"=-158.89802683480974}, {"X"=398000.0, "Y"=-158.95255872770184}, {"X"=399000.0, "Y"=-159.00680377083165}, {"X"=400000.0, "Y"=-159.06076423687176}, {"X"=401000.0, "Y"=-159.11444237452736}, {"X"=402000.0, "Y"=-159.1678404088692}, {"X"=403000.0, "Y"=-159.2209605416285}, {"X"=404000.0, "Y"=-159.2738049515071}, {"X"=405000.0, "Y"=-159.3263757944766}, {"X"=406000.0, "Y"=-159.37867520407144}, {"X"=407000.0, "Y"=-159.43070529169108}, {"X"=408000.0, "Y"=-159.482468146868}, {"X"=409000.0, "Y"=-159.5339658375603}, {"X"=410000.0, "Y"=-159.5852004104284}, {"X"=411000.0, "Y"=-159.6361738911096}, {"X"=412000.0, "Y"=-159.68688828447802}, {"X"=413000.0, "Y"=-159.73734557492506}, {"X"=414000.0, "Y"=-159.78754772660267}, {"X"=415000.0, "Y"=-159.83749668369938}, {"X"=416000.0, "Y"=-159.88719437067056}, {"X"=417000.0, "Y"=-159.93664269251192}, {"X"=418000.0, "Y"=-159.9858435349849}, {"X"=419000.0, "Y"=-160.0347987648709}, {"X"=420000.0, "Y"=-160.08351023020543}, {"X"=421000.0, "Y"=-160.13197976050844}, {"X"=422000.0, "Y"=-160.18020916702156}, {"X"=423000.0, "Y"=-160.22820024293833}, {"X"=424000.0, "Y"=-160.27595476361452}, {"X"=425000.0, "Y"=-160.32347448680687}, {"X"=426000.0, "Y"=-160.37076115287618}, {"X"=427000.0, "Y"=-160.4178164850082}, {"X"=428000.0, "Y"=-160.4646421894294}, {"X"=429000.0, "Y"=-160.51123995560505}, {"X"=430000.0, "Y"=-160.55761145644547}, {"X"=431000.0, "Y"=-160.60375834852044}, {"X"=432000.0, "Y"=-160.64968227224307}, {"X"=433000.0, "Y"=-160.69538485207534}, {"X"=434000.0, "Y"=-160.74086769671902}, {"X"=435000.0, "Y"=-160.7861323993011}, {"X"=436000.0, "Y"=-160.83118053757246}, {"X"=437000.0, "Y"=-160.87601367408234}, {"X"=438000.0, "Y"=-160.920633356371}, {"X"=439000.0, "Y"=-160.9650411171329}, {"X"=440000.0, "Y"=-161.00923847441427}, {"X"=441000.0, "Y"=-161.05322693177004}, {"X"=442000.0, "Y"=-161.09700797845233}, {"X"=443000.0, "Y"=-161.14058308956444}, {"X"=444000.0, "Y"=-161.183953726237}, {"X"=445000.0, "Y"=-161.22712133579535}, {"X"=446000.0, "Y"=-161.27008735191376}, {"X"=447000.0, "Y"=-161.31285319477695}, {"X"=448000.0, "Y"=-161.3554202712443}, {"X"=449000.0, "Y"=-161.39778997500204}, {"X"=450000.0, "Y"=-161.439963686717}, {"X"=451000.0, "Y"=-161.48194277418781}, {"X"=452000.0, "Y"=-161.52372859249058}, {"X"=453000.0, "Y"=-161.5653224841365}, {"X"=454000.0, "Y"=-161.60672577920354}, {"X"=455000.0, "Y"=-161.64793979548784}, {"X"=456000.0, "Y"=-161.68896583864483}, {"X"=457000.0, "Y"=-161.729805202328}, {"X"=458000.0, "Y"=-161.77045916831574}, {"X"=459000.0, "Y"=-161.8109290066671}, {"X"=460000.0, "Y"=-161.8512159758386}, {"X"=461000.0, "Y"=-161.89132132281918}, {"X"=462000.0, "Y"=-161.93124628327007}, {"X"=463000.0, "Y"=-161.9709920816315}, {"X"=464000.0, "Y"=-162.01055993127935}, {"X"=465000.0, "Y"=-162.04995103461482}, {"X"=466000.0, "Y"=-162.08916658322414}, {"X"=467000.0, "Y"=-162.12820775796246}, {"X"=468000.0, "Y"=-162.16707572910752}, {"X"=469000.0, "Y"=-162.2057716564517}, {"X"=470000.0, "Y"=-162.24429668943264}, {"X"=471000.0, "Y"=-162.28265196724772}, {"X"=472000.0, "Y"=-162.3208386189596}, {"X"=473000.0, "Y"=-162.35885776361266}, {"X"=474000.0, "Y"=-162.3967105103484}, {"X"=475000.0, "Y"=-162.43439795850094}, {"X"=476000.0, "Y"=-162.47192119771972}, {"X"=477000.0, "Y"=-162.50928130806454}, {"X"=478000.0, "Y"=-162.54647936011628}, {"X"=479000.0, "Y"=-162.58351641507426}, {"X"=480000.0, "Y"=-162.62039352486784}, {"X"=481000.0, "Y"=-162.65711173224173}, {"X"=482000.0, "Y"=-162.69367207087436}, {"X"=483000.0, "Y"=-162.73007556545554}, {"X"=484000.0, "Y"=-162.76632323180462}, {"X"=485000.0, "Y"=-162.8024160769425}, {"X"=486000.0, "Y"=-162.83835509920715}, {"X"=487000.0, "Y"=-162.8741412883345}, {"X"=488000.0, "Y"=-162.90977562554733}, {"X"=489000.0, "Y"=-162.94525908365762}, {"X"=490000.0, "Y"=-162.98059262715032}, {"X"=491000.0, "Y"=-163.01577721226818}, {"X"=492000.0, "Y"=-163.05081378709912}, {"X"=493000.0, "Y"=-163.08570329167014}, {"X"=494000.0, "Y"=-163.1204466580244}, {"X"=495000.0, "Y"=-163.15504481030632}, {"X"=496000.0, "Y"=-163.1894986648462}, {"X"=497000.0, "Y"=-163.22380913024173}, {"X"=498000.0, "Y"=-163.25797710744118}, {"X"=499000.0, "Y"=-163.29200348981553}, {"X"=500000.0, "Y"=-163.32588916324346}, {"X"=501000.0, "Y"=-163.35963500618743}, {"X"=502000.0, "Y"=-163.39324188977304}, {"X"=503000.0, "Y"=-163.42671067785352}, {"X"=504000.0, "Y"=-163.4600422271063}, {"X"=505000.0, "Y"=-163.49323738708432}, {"X"=506000.0, "Y"=-163.5262970002999}, {"X"=507000.0, "Y"=-163.5592219022998}, {"X"=508000.0, "Y"=-163.59201292172673}, {"X"=509000.0, "Y"=-163.62467088039767}, {"X"=510000.0, "Y"=-163.65719659337321}, {"X"=511000.0, "Y"=-163.68959086901728}, {"X"=512000.0, "Y"=-163.72185450908026}, {"X"=513000.0, "Y"=-163.75398830874775}, {"X"=514000.0, "Y"=-163.7859930567251}, {"X"=515000.0, "Y"=-163.81786953528342}, {"X"=516000.0, "Y"=-163.84961852034616}, {"X"=517000.0, "Y"=-163.8812407815348}, {"X"=518000.0, "Y"=-163.91273708223645}, {"X"=519000.0, "Y"=-163.94410817967233}, {"X"=520000.0, "Y"=-163.97535482495294}, {"X"=521000.0, "Y"=-164.00647776314057}, {"X"=522000.0, "Y"=-164.03747773331463}, {"X"=523000.0, "Y"=-164.06835546861464}, {"X"=524000.0, "Y"=-164.099111696325}, {"X"=525000.0, "Y"=-164.12974713790615}, {"X"=526000.0, "Y"=-164.16026250906873}, {"X"=527000.0, "Y"=-164.19065851983063}, {"X"=528000.0, "Y"=-164.22093587455512}, {"X"=529000.0, "Y"=-164.25109527203134}, {"X"=530000.0, "Y"=-164.28113740550998}, {"X"=531000.0, "Y"=-164.3110629627629}, {"X"=532000.0, "Y"=-164.3408726261439}, {"X"=533000.0, "Y"=-164.37056707262474}, {"X"=534000.0, "Y"=-164.4001469738671}, {"X"=535000.0, "Y"=-164.42961299625824}, {"X"=536000.0, "Y"=-164.4589658009713}, {"X"=537000.0, "Y"=-164.4882060440089}, {"X"=538000.0, "Y"=-164.5173343762627}, {"X"=539000.0, "Y"=-164.5463514435508}, {"X"=540000.0, "Y"=-164.57525788667465}, {"X"=541000.0, "Y"=-164.60405434146077}, {"X"=542000.0, "Y"=-164.63274143882057}, {"X"=543000.0, "Y"=-164.66131980478065}, {"X"=544000.0, "Y"=-164.6897900605403}, {"X"=545000.0, "Y"=-164.718152822518}, {"X"=546000.0, "Y"=-164.7464087023889}, {"X"=547000.0, "Y"=-164.77455830713404}, {"X"=548000.0, "Y"=-164.802602239091}, {"X"=549000.0, "Y"=-164.83054109598473}, {"X"=550000.0, "Y"=-164.85837547098592}, {"X"=551000.0, "Y"=-164.88610595273775}, {"X"=552000.0, "Y"=-164.9137331254148}, {"X"=553000.0, "Y"=-164.94125756875192}, {"X"=554000.0, "Y"=-164.9686798580936}, {"X"=555000.0, "Y"=-164.99600056443313}, {"X"=556000.0, "Y"=-165.02322025444983}, {"X"=557000.0, "Y"=-165.050339490555}, {"X"=558000.0, "Y"=-165.07735883092738}, {"X"=559000.0, "Y"=-165.10427882955273}, {"X"=560000.0, "Y"=-165.13110003626508}, {"X"=561000.0, "Y"=-165.15782299678352}, {"X"=562000.0, "Y"=-165.18444825275287}, {"X"=563000.0, "Y"=-165.2109763417742}, {"X"=564000.0, "Y"=-165.23740779745242}, {"X"=565000.0, "Y"=-165.26374314942314}, {"X"=566000.0, "Y"=-165.28998292339634}, {"X"=567000.0, "Y"=-165.31612764118722}, {"X"=568000.0, "Y"=-165.34217782075595}, {"X"=569000.0, "Y"=-165.3681339762423}, {"X"=570000.0, "Y"=-165.3939966179973}, {"X"=571000.0, "Y"=-165.41976625261952}, {"X"=572000.0, "Y"=-165.44544338299343}, {"X"=573000.0, "Y"=-165.4710285083126}, {"X"=574000.0, "Y"=-165.49652212412863}, {"X"=575000.0, "Y"=-165.5219247223668}, {"X"=576000.0, "Y"=-165.54723679137203}, {"X"=577000.0, "Y"=-165.5724588159398}, {"X"=578000.0, "Y"=-165.597591277336}, {"X"=579000.0, "Y"=-165.6226346533458}, {"X"=580000.0, "Y"=-165.6475894182951}, {"X"=581000.0, "Y"=-165.67245604307925}, {"X"=582000.0, "Y"=-165.697234995203}, {"X"=583000.0, "Y"=-165.7219267388062}, {"X"=584000.0, "Y"=-165.74653173468394}, {"X"=585000.0, "Y"=-165.77105044034096}, {"X"=586000.0, "Y"=-165.795483309992}, {"X"=587000.0, "Y"=-165.81983079461384}, {"X"=588000.0, "Y"=-165.84409334195925}, {"X"=589000.0, "Y"=-165.8682713965988}, {"X"=590000.0, "Y"=-165.892365399934}, {"X"=591000.0, "Y"=-165.91637579023842}, {"X"=592000.0, "Y"=-165.94030300267616}, {"X"=593000.0, "Y"=-165.9641474693366}, {"X"=594000.0, "Y"=-165.98790961925698}, {"X"=595000.0, "Y"=-166.0115898784473}, {"X"=596000.0, "Y"=-166.03518866992636}, {"X"=597000.0, "Y"=-166.05870641373372}, {"X"=598000.0, "Y"=-166.08214352697075}, {"X"=599000.0, "Y"=-166.10550042381306}, {"X"=600000.0, "Y"=-166.12877751554623}, {"X"=601000.0, "Y"=-166.15197521058877}, {"X"=602000.0, "Y"=-166.175093914507}, {"X"=603000.0, "Y"=-166.1981340300556}, {"X"=604000.0, "Y"=-166.22109595719553}, {"X"=605000.0, "Y"=-166.24398009310994}, {"X"=606000.0, "Y"=-166.26678683224173}, {"X"=607000.0, "Y"=-166.2895165663104}, {"X"=608000.0, "Y"=-166.31216968433438}, {"X"=609000.0, "Y"=-166.33474657265685}, {"X"=610000.0, "Y"=-166.35724761496914}, {"X"=611000.0, "Y"=-166.37967319233206}, {"X"=612000.0, "Y"=-166.40202368319808}, {"X"=613000.0, "Y"=-166.42429946343833}, {"X"=614000.0, "Y"=-166.4465009063532}, {"X"=615000.0, "Y"=-166.46862838271602}, {"X"=616000.0, "Y"=-166.49068226076542}, {"X"=617000.0, "Y"=-166.51266290625108}, {"X"=618000.0, "Y"=-166.5345706824442}, {"X"=619000.0, "Y"=-166.5564059501633}, {"X"=620000.0, "Y"=-166.57816906778868}, {"X"=621000.0, "Y"=-166.59986039128881}, {"X"=622000.0, "Y"=-166.62148027423876}, {"X"=623000.0, "Y"=-166.64302906783865}, {"X"=624000.0, "Y"=-166.66450712094047}, {"X"=625000.0, "Y"=-166.68591478005737}, {"X"=626000.0, "Y"=-166.70725238939588}, {"X"=627000.0, "Y"=-166.7285202908596}, {"X"=628000.0, "Y"=-166.74971882408693}, {"X"=629000.0, "Y"=-166.77084832645193}, {"X"=630000.0, "Y"=-166.7919091331034}, {"X"=631000.0, "Y"=-166.812901576959}, {"X"=632000.0, "Y"=-166.83382598874692}, {"X"=633000.0, "Y"=-166.85468269701005}, {"X"=634000.0, "Y"=-166.8754720281326}, {"X"=635000.0, "Y"=-166.89619430634912}, {"X"=636000.0, "Y"=-166.91684985377026}, {"X"=637000.0, "Y"=-166.9374389903969}, {"X"=638000.0, "Y"=-166.9579620341388}, {"X"=639000.0, "Y"=-166.97841930083342}, {"X"=640000.0, "Y"=-166.99881110425645}, {"X"=641000.0, "Y"=-167.01913775614793}, {"X"=642000.0, "Y"=-167.03939956622395}, {"X"=643000.0, "Y"=-167.0595968421901}, {"X"=644000.0, "Y"=-167.0797298897691}, {"X"=645000.0, "Y"=-167.09979901270708}, {"X"=646000.0, "Y"=-167.11980451278782}, {"X"=647000.0, "Y"=-167.13974668986202}, {"X"=648000.0, "Y"=-167.1596258418498}, {"X"=649000.0, "Y"=-167.17944226476368}, {"X"=650000.0, "Y"=-167.19919625272428}, {"X"=651000.0, "Y"=-167.21888809797076}, {"X"=652000.0, "Y"=-167.23851809087813}, {"X"=653000.0, "Y"=-167.2580865199779}, {"X"=654000.0, "Y"=-167.2775936719642}, {"X"=655000.0, "Y"=-167.29703983171515}, {"X"=656000.0, "Y"=-167.31642528230861}, {"X"=657000.0, "Y"=-167.33575030502857}, {"X"=658000.0, "Y"=-167.35501517938872}, {"X"=659000.0, "Y"=-167.37422018314032}, {"X"=660000.0, "Y"=-167.3933655922882}, {"X"=661000.0, "Y"=-167.4124516811126}, {"X"=662000.0, "Y"=-167.43147872216855}, {"X"=663000.0, "Y"=-167.4504469863134}, {"X"=664000.0, "Y"=-167.469356742708}, {"X"=665000.0, "Y"=-167.48820825884087}, {"X"=666000.0, "Y"=-167.5070018005389}, {"X"=667000.0, "Y"=-167.52573763197432}, {"X"=668000.0, "Y"=-167.54441601568874}, {"X"=669000.0, "Y"=-167.56303721259638}, {"X"=670000.0, "Y"=-167.58160148200147}, {"X"=671000.0, "Y"=-167.60010908161064}, {"X"=672000.0, "Y"=-167.61856026754742}, {"X"=673000.0, "Y"=-167.63695529436018}, {"X"=674000.0, "Y"=-167.65529441504094}, {"X"=675000.0, "Y"=-167.67357788103067}, {"X"=676000.0, "Y"=-167.69180594223417}, {"X"=677000.0, "Y"=-167.70997884704002}, {"X"=678000.0, "Y"=-167.72809684231584}, {"X"=679000.0, "Y"=-167.74616017344022}, {"X"=680000.0, "Y"=-167.7641690842944}, {"X"=681000.0, "Y"=-167.78212381729122}, {"X"=682000.0, "Y"=-167.80002461337756}, {"X"=683000.0, "Y"=-167.8178717120461}, {"X"=684000.0, "Y"=-167.83566535134867}, {"X"=685000.0, "Y"=-167.85340576790622}, {"X"=686000.0, "Y"=-167.87109319692496}, {"X"=687000.0, "Y"=-167.88872787219867}, {"X"=688000.0, "Y"=-167.90631002612452}, {"X"=689000.0, "Y"=-167.92383988971835}, {"X"=690000.0, "Y"=-167.9413176926172}, {"X"=691000.0, "Y"=-167.9587436630913}, {"X"=692000.0, "Y"=-167.97611802806352}, {"X"=693000.0, "Y"=-167.9934410131063}, {"X"=694000.0, "Y"=-168.01071284246473}, {"X"=695000.0, "Y"=-168.02793373905615}, {"X"=696000.0, "Y"=-168.04510392448788}, {"X"=697000.0, "Y"=-168.06222361906606}, {"X"=698000.0, "Y"=-168.0792930418005}, {"X"=699000.0, "Y"=-168.09631241042445}, {"X"=700000.0, "Y"=-168.11328194138963}, {"X"=701000.0, "Y"=-168.13020184989165}, {"X"=702000.0, "Y"=-168.14707234987446}, {"X"=703000.0, "Y"=-168.16389365402836}, {"X"=704000.0, "Y"=-168.18066597382034}, {"X"=705000.0, "Y"=-168.19738951948756}, {"X"=706000.0, "Y"=-168.2140645000468}, {"X"=707000.0, "Y"=-168.23069112332047}, {"X"=708000.0, "Y"=-168.24726959591976}, {"X"=709000.0, "Y"=-168.26380012327962}, {"X"=710000.0, "Y"=-168.2802829096496}, {"X"=711000.0, "Y"=-168.2967181581093}, {"X"=712000.0, "Y"=-168.31310607057924}, {"X"=713000.0, "Y"=-168.32944684782456}, {"X"=714000.0, "Y"=-168.34574068946642}, {"X"=715000.0, "Y"=-168.36198779399518}, {"X"=716000.0, "Y"=-168.37818835876612}, {"X"=717000.0, "Y"=-168.39434258002626}, {"X"=718000.0, "Y"=-168.41045065290166}, {"X"=719000.0, "Y"=-168.42651277142443}, {"X"=720000.0, "Y"=-168.44252912853074}, {"X"=721000.0, "Y"=-168.45849991606832}, {"X"=722000.0, "Y"=-168.47442532481347}, {"X"=723000.0, "Y"=-168.49030554446574}, {"X"=724000.0, "Y"=-168.50614076367145}, {"X"=725000.0, "Y"=-168.52193117001553}, {"X"=726000.0, "Y"=-168.53767695004058}, {"X"=727000.0, "Y"=-168.55337828925167}, {"X"=728000.0, "Y"=-168.56903537212276}, {"X"=729000.0, "Y"=-168.5846483821042}, {"X"=730000.0, "Y"=-168.60021750163077}, {"X"=731000.0, "Y"=-168.61574291213236}, {"X"=732000.0, "Y"=-168.63122479403518}, {"X"=733000.0, "Y"=-168.64666332677018}, {"X"=734000.0, "Y"=-168.66205868878745}, {"X"=735000.0, "Y"=-168.67741105755613}, {"X"=736000.0, "Y"=-168.69272060957184}, {"X"=737000.0, "Y"=-168.7079875203679}, {"X"=738000.0, "Y"=-168.7232119645202}, {"X"=739000.0, "Y"=-168.738394115652}, {"X"=740000.0, "Y"=-168.75353414644508}, {"X"=741000.0, "Y"=-168.768632228642}, {"X"=742000.0, "Y"=-168.78368853305636}, {"X"=743000.0, "Y"=-168.79870322957896}, {"X"=744000.0, "Y"=-168.8136764871826}, {"X"=745000.0, "Y"=-168.82860847392885}, {"X"=746000.0, "Y"=-168.84349935697867}, {"X"=747000.0, "Y"=-168.85834930259352}, {"X"=748000.0, "Y"=-168.87315847614434}, {"X"=749000.0, "Y"=-168.88792704211778}, {"X"=750000.0, "Y"=-168.90265516412154}, {"X"=751000.0, "Y"=-168.91734300489344}, {"X"=752000.0, "Y"=-168.93199072630347}, {"X"=753000.0, "Y"=-168.9465984893618}, {"X"=754000.0, "Y"=-168.96116645422939}, {"X"=755000.0, "Y"=-168.97569478021433}, {"X"=756000.0, "Y"=-168.99018362578636}, {"X"=757000.0, "Y"=-169.00463314857672}, {"X"=758000.0, "Y"=-169.01904350539053}, {"X"=759000.0, "Y"=-169.0334148522099}, {"X"=760000.0, "Y"=-169.04774734419266}, {"X"=761000.0, "Y"=-169.0620411356901}, {"X"=762000.0, "Y"=-169.0762963802477}, {"X"=763000.0, "Y"=-169.0905132306026}, {"X"=764000.0, "Y"=-169.1046918387068}, {"X"=765000.0, "Y"=-169.1188323557115}, {"X"=766000.0, "Y"=-169.13293493199257}, {"X"=767000.0, "Y"=-169.14699971714447}, {"X"=768000.0, "Y"=-169.1610268599834}, {"X"=769000.0, "Y"=-169.17501650856525}, {"X"=770000.0, "Y"=-169.188968810174}, {"X"=771000.0, "Y"=-169.20288391134596}, {"X"=772000.0, "Y"=-169.21676195785653}, {"X"=773000.0, "Y"=-169.23060309473954}, {"X"=774000.0, "Y"=-169.24440746628443}, {"X"=775000.0, "Y"=-169.25817521604336}, {"X"=776000.0, "Y"=-169.27190648683523}, {"X"=777000.0, "Y"=-169.28560142075662}, {"X"=778000.0, "Y"=-169.29926015917982}, {"X"=779000.0, "Y"=-169.3128828427549}, {"X"=780000.0, "Y"=-169.32646961142933}, {"X"=781000.0, "Y"=-169.34002060443464}, {"X"=782000.0, "Y"=-169.35353596030552}, {"X"=783000.0, "Y"=-169.36701581687515}, {"X"=784000.0, "Y"=-169.38046031128653}, {"X"=785000.0, "Y"=-169.39386957998897}, {"X"=786000.0, "Y"=-169.40724375875487}, {"X"=787000.0, "Y"=-169.4205829826737}, {"X"=788000.0, "Y"=-169.43388738616068}, {"X"=789000.0, "Y"=-169.44715710295975}, {"X"=790000.0, "Y"=-169.46039226615073}, {"X"=791000.0, "Y"=-169.47359300815037}, {"X"=792000.0, "Y"=-169.48675946072132}, {"X"=793000.0, "Y"=-169.49989175497342}, {"X"=794000.0, "Y"=-169.51299002136432}, {"X"=795000.0, "Y"=-169.52605438971102}, {"X"=796000.0, "Y"=-169.53908498919344}, {"X"=797000.0, "Y"=-169.55208194834938}, {"X"=798000.0, "Y"=-169.56504539509393}, {"X"=799000.0, "Y"=-169.57797545670513}, {"X"=800000.0, "Y"=-169.5908722598462}, {"X"=801000.0, "Y"=-169.60373593055988}, {"X"=802000.0, "Y"=-169.61656659427}, {"X"=803000.0, "Y"=-169.62936437579532}, {"X"=804000.0, "Y"=-169.64212939934157}, {"X"=805000.0, "Y"=-169.6548617885178}, {"X"=806000.0, "Y"=-169.66756166633195}, {"X"=807000.0, "Y"=-169.68022915519447}, {"X"=808000.0, "Y"=-169.69286437692807}, {"X"=809000.0, "Y"=-169.70546745276442}, {"X"=810000.0, "Y"=-169.71803850335579}, {"X"=811000.0, "Y"=-169.7305776487707}, {"X"=812000.0, "Y"=-169.7430850085044}, {"X"=813000.0, "Y"=-169.75556070148082}, {"X"=814000.0, "Y"=-169.7680048460495}, {"X"=815000.0, "Y"=-169.78041755999965}, {"X"=816000.0, "Y"=-169.79279896055868}, {"X"=817000.0, "Y"=-169.8051491643946}, {"X"=818000.0, "Y"=-169.81746828762277}, {"X"=819000.0, "Y"=-169.82975644580324}, {"X"=820000.0, "Y"=-169.84201375395565}, {"X"=821000.0, "Y"=-169.85424032655112}, {"X"=822000.0, "Y"=-169.86643627752005}, {"X"=823000.0, "Y"=-169.87860172026046}, {"X"=824000.0, "Y"=-169.89073676763036}, {"X"=825000.0, "Y"=-169.90284153196086}, {"X"=826000.0, "Y"=-169.91491612505513}, {"X"=827000.0, "Y"=-169.92696065819644}, {"X"=828000.0, "Y"=-169.93897524214094}, {"X"=829000.0, "Y"=-169.9509599871326}, {"X"=830000.0, "Y"=-169.962915002898}, {"X"=831000.0, "Y"=-169.97484039865935}, {"X"=832000.0, "Y"=-169.98673628312167}, {"X"=833000.0, "Y"=-169.99860276449527}, {"X"=834000.0, "Y"=-170.01043995048025}, {"X"=835000.0, "Y"=-170.02224794828527}, {"X"=836000.0, "Y"=-170.03402686461982}, {"X"=837000.0, "Y"=-170.04577680570424}, {"X"=838000.0, "Y"=-170.05749787726654}, {"X"=839000.0, "Y"=-170.06919018455187}, {"X"=840000.0, "Y"=-170.0808538323214}, {"X"=841000.0, "Y"=-170.09248892485323}, {"X"=842000.0, "Y"=-170.10409556595158}, {"X"=843000.0, "Y"=-170.1156738589438}, {"X"=844000.0, "Y"=-170.1272239066887}, {"X"=845000.0, "Y"=-170.13874581157273}, {"X"=846000.0, "Y"=-170.15023967551957}, {"X"=847000.0, "Y"=-170.16170559999085}, {"X"=848000.0, "Y"=-170.1731436859829}, {"X"=849000.0, "Y"=-170.18455403404153}, {"X"=850000.0, "Y"=-170.19593674424914}, {"X"=851000.0, "Y"=-170.20729191624451}, {"X"=852000.0, "Y"=-170.21861964921095}, {"X"=853000.0, "Y"=-170.22992004189342}, {"X"=854000.0, "Y"=-170.24119319258182}, {"X"=855000.0, "Y"=-170.2524391991334}, {"X"=856000.0, "Y"=-170.26365815895963}, {"X"=857000.0, "Y"=-170.2748501690482}, {"X"=858000.0, "Y"=-170.28601532593666}, {"X"=859000.0, "Y"=-170.29715372574492}, {"X"=860000.0, "Y"=-170.30826546415688}, {"X"=861000.0, "Y"=-170.31935063643624}, {"X"=862000.0, "Y"=-170.3304093374203}, {"X"=863000.0, "Y"=-170.34144166152151}, {"X"=864000.0, "Y"=-170.35244770274318}, {"X"=865000.0, "Y"=-170.3634275546624}, {"X"=866000.0, "Y"=-170.3743813104511}, {"X"=867000.0, "Y"=-170.3853090628662}, {"X"=868000.0, "Y"=-170.39621090425567}, {"X"=869000.0, "Y"=-170.4070869265604}, {"X"=870000.0, "Y"=-170.41793722132041}, {"X"=871000.0, "Y"=-170.42876187966988}, {"X"=872000.0, "Y"=-170.43956099234845}, {"X"=873000.0, "Y"=-170.45033464969288}, {"X"=874000.0, "Y"=-170.46108294165015}, {"X"=875000.0, "Y"=-170.47180595777144}, {"X"=876000.0, "Y"=-170.4825037872193}, {"X"=877000.0, "Y"=-170.49317651876515}, {"X"=878000.0, "Y"=-170.5038242408017}, {"X"=879000.0, "Y"=-170.51444704132808}, {"X"=880000.0, "Y"=-170.52504500796897}, {"X"=881000.0, "Y"=-170.53561822796797}, {"X"=882000.0, "Y"=-170.54616678819127}, {"X"=883000.0, "Y"=-170.55669077512897}, {"X"=884000.0, "Y"=-170.56719027489828}, {"X"=885000.0, "Y"=-170.57766537324778}, {"X"=886000.0, "Y"=-170.5881161555542}, {"X"=887000.0, "Y"=-170.5985427068295}, {"X"=888000.0, "Y"=-170.60894511172205}, {"X"=889000.0, "Y"=-170.61932345451373}, {"X"=890000.0, "Y"=-170.62967781912857}, {"X"=891000.0, "Y"=-170.64000828913055}, {"X"=892000.0, "Y"=-170.6503149477287}, {"X"=893000.0, "Y"=-170.6605978777763}, {"X"=894000.0, "Y"=-170.6708571617732}, {"X"=895000.0, "Y"=-170.68109288187014}, {"X"=896000.0, "Y"=-170.6913051198668}, {"X"=897000.0, "Y"=-170.70149395722092}, {"X"=898000.0, "Y"=-170.7116594750379}, {"X"=899000.0, "Y"=-170.721801754083}, {"X"=900000.0, "Y"=-170.73192087478463}, {"X"=901000.0, "Y"=-170.74201691722698}, {"X"=902000.0, "Y"=-170.75208996115583}, {"X"=903000.0, "Y"=-170.7621400859843}, {"X"=904000.0, "Y"=-170.77216737079107}, {"X"=905000.0, "Y"=-170.78217189432257}, {"X"=906000.0, "Y"=-170.79215373499312}, {"X"=907000.0, "Y"=-170.80211297089028}, {"X"=908000.0, "Y"=-170.81204967977595}, {"X"=909000.0, "Y"=-170.82196393908345}, {"X"=910000.0, "Y"=-170.8318558259266}, {"X"=911000.0, "Y"=-170.8417254170975}, {"X"=912000.0, "Y"=-170.85157278906485}, {"X"=913000.0, "Y"=-170.86139801798197}, {"X"=914000.0, "Y"=-170.87120117968527}, {"X"=915000.0, "Y"=-170.88098234969868}, {"X"=916000.0, "Y"=-170.8907416032265}, {"X"=917000.0, "Y"=-170.9004790151714}, {"X"=918000.0, "Y"=-170.9101946601187}, {"X"=919000.0, "Y"=-170.9198886123479}, {"X"=920000.0, "Y"=-170.92956094583292}, {"X"=921000.0, "Y"=-170.9392117342399}, {"X"=922000.0, "Y"=-170.94884105093666}, {"X"=923000.0, "Y"=-170.95844896898512}, {"X"=924000.0, "Y"=-170.968035561149}, {"X"=925000.0, "Y"=-170.9776008998923}, {"X"=926000.0, "Y"=-170.9871450573835}, {"X"=927000.0, "Y"=-170.99666810549434}, {"X"=928000.0, "Y"=-171.00617011580306}, {"X"=929000.0, "Y"=-171.01565115959846}, {"X"=930000.0, "Y"=-171.02511130786934}, {"X"=931000.0, "Y"=-171.034550631329}, {"X"=932000.0, "Y"=-171.04396920039255}, {"X"=933000.0, "Y"=-171.05336708519104}, {"X"=934000.0, "Y"=-171.0627443555726}, {"X"=935000.0, "Y"=-171.07210108109888}, {"X"=936000.0, "Y"=-171.08143733105157}, {"X"=937000.0, "Y"=-171.09075317443006}, {"X"=938000.0, "Y"=-171.1000486799598}, {"X"=939000.0, "Y"=-171.10932391608083}, {"X"=940000.0, "Y"=-171.11857895096307}, {"X"=941000.0, "Y"=-171.12781385249878}, {"X"=942000.0, "Y"=-171.1370286883074}, {"X"=943000.0, "Y"=-171.1462235257357}, {"X"=944000.0, "Y"=-171.15539843186104}, {"X"=945000.0, "Y"=-171.16455347348693}, {"X"=946000.0, "Y"=-171.1736887171586}, {"X"=947000.0, "Y"=-171.18280422914245}, {"X"=948000.0, "Y"=-171.1919000754492}, {"X"=949000.0, "Y"=-171.20097632182035}, {"X"=950000.0, "Y"=-171.210033033736}, {"X"=951000.0, "Y"=-171.2190702764147}, {"X"=952000.0, "Y"=-171.22808811481787}, {"X"=953000.0, "Y"=-171.23708661364424}, {"X"=954000.0, "Y"=-171.24606583733322}, {"X"=955000.0, "Y"=-171.25502585007683}, {"X"=956000.0, "Y"=-171.26396671580284}, {"X"=957000.0, "Y"=-171.27288849819024}, {"X"=958000.0, "Y"=-171.2817912606635}, {"X"=959000.0, "Y"=-171.29067506639632}, {"X"=960000.0, "Y"=-171.29953997831353}, {"X"=961000.0, "Y"=-171.30838605909224}, {"X"=962000.0, "Y"=-171.3172133711563}, {"X"=963000.0, "Y"=-171.32602197668905}, {"X"=964000.0, "Y"=-171.33481193762987}, {"X"=965000.0, "Y"=-171.34358331566784}, {"X"=966000.0, "Y"=-171.35233617225066}, {"X"=967000.0, "Y"=-171.36107056859174}, {"X"=968000.0, "Y"=-171.36978656565344}, {"X"=969000.0, "Y"=-171.37848422416812}, {"X"=970000.0, "Y"=-171.3871636046261}, {"X"=971000.0, "Y"=-171.39582476727946}, {"X"=972000.0, "Y"=-171.40446777214515}, {"X"=973000.0, "Y"=-171.41309267900937}, {"X"=974000.0, "Y"=-171.42169954741922}, {"X"=975000.0, "Y"=-171.4302884366906}, {"X"=976000.0, "Y"=-171.43885940591395}, {"X"=977000.0, "Y"=-171.44741251394066}, {"X"=978000.0, "Y"=-171.45594781939792}, {"X"=979000.0, "Y"=-171.46446538068824}, {"X"=980000.0, "Y"=-171.47296525597795}, {"X"=981000.0, "Y"=-171.48144750321592}, {"X"=982000.0, "Y"=-171.48991218012208}, {"X"=983000.0, "Y"=-171.49835934419633}, {"X"=984000.0, "Y"=-171.5067890527078}, {"X"=985000.0, "Y"=-171.51520136271483}, {"X"=986000.0, "Y"=-171.52359633104857}, {"X"=987000.0, "Y"=-171.53197401431896}, {"X"=988000.0, "Y"=-171.54033446892674}, {"X"=989000.0, "Y"=-171.54867775104316}, {"X"=990000.0, "Y"=-171.55700391663225}, {"X"=991000.0, "Y"=-171.56531302143458}, {"X"=992000.0, "Y"=-171.57360512098694}, {"X"=993000.0, "Y"=-171.58188027060555}, {"X"=994000.0, "Y"=-171.59013852539033}, {"X"=995000.0, "Y"=-171.59837994023974}, {"X"=996000.0, "Y"=-171.60660456983345}, {"X"=997000.0, "Y"=-171.61481246864776}, {"X"=998000.0, "Y"=-171.6230036909456}, {"X"=999000.0, "Y"=-171.6311782907842}, {"X"=1000000.0, "Y"=-171.63933632201622}]
  # "Measurement Configuration"
  # "Filter Configuration"
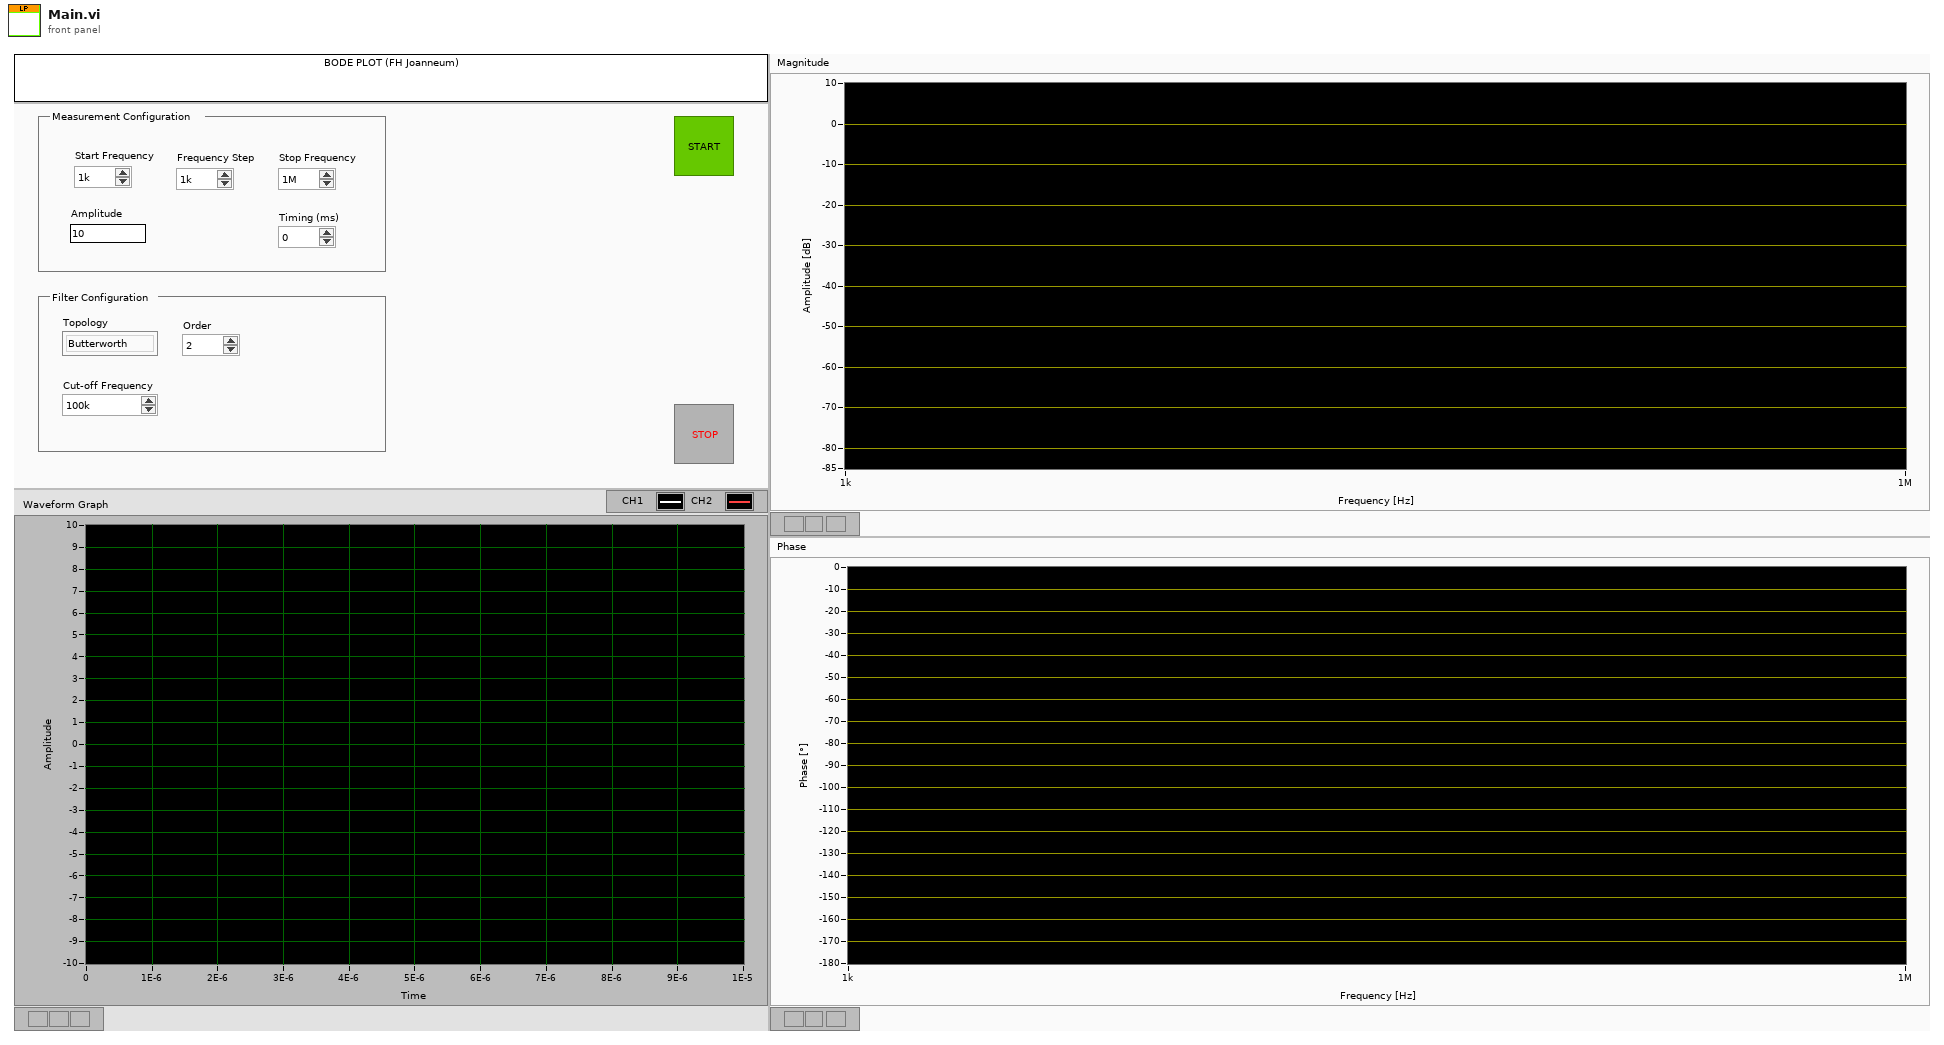
[diagram p1: front panel]
types:
  T1 = enum16{"Off", "Butterworth", "Chebyshev", "Inverse Chebyshev", "Elliptic", "Bessel"}
  T2 = cluster{"Settings":cluster{"f":dbl, "Start Freq.":dbl, "Freq. Step":dbl, "Stop Frequ.":dbl, "Amplitude":dbl, "Calculated":cluster{"Amplitude":cluster{"X":dbl, "Y":dbl}[], "Phase":cluster{"X":dbl, "Y":dbl}[]}}, "Acquired":cluster{"Input":waveform(dbl), "Output":waveform(dbl)}}
  T3 = enum16{"Lowpass", "Highpass", "Bandpass", "Bandstop"}
  T4 = cluster{"Topology":enum16{"Off", "Butterworth", "Chebyshev", "Inverse Chebyshev", "Elliptic", "Bessel"}, "Type":enum16{"Lowpass", "Highpass", "Bandpass", "Bandstop"}, "Order":i32, "Lower Fc":dbl, "Upper Fc":dbl, "PB Ripple":dbl, "SB Attenuation":dbl}
  T5 = enum32{"none", "input signal", "detected signal", "residual signal"}
  T6 = cluster{"Amplitude":cluster{"X":dbl, "Y":dbl}[], "Phase":cluster{"X":dbl, "Y":dbl}[]}
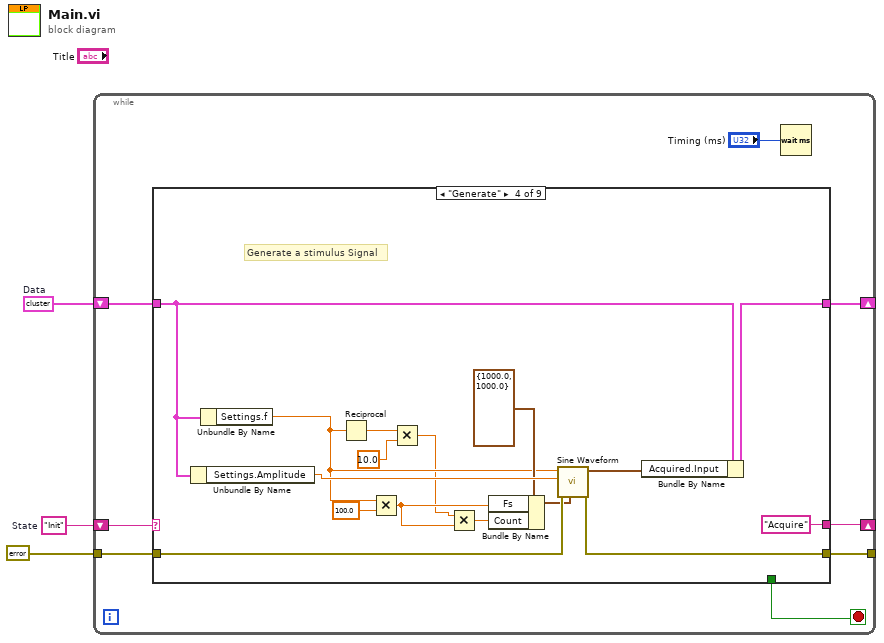
[diagram p0: block diagram]
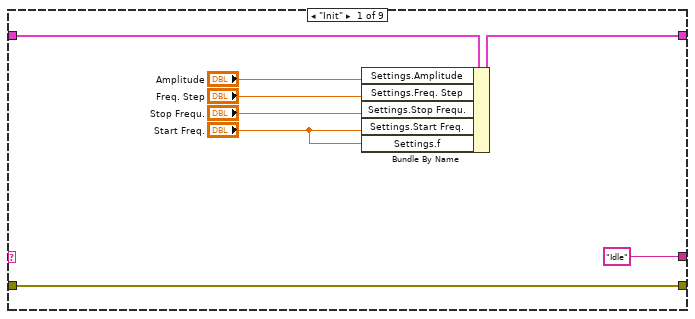
[diagram p2: hidden frame]
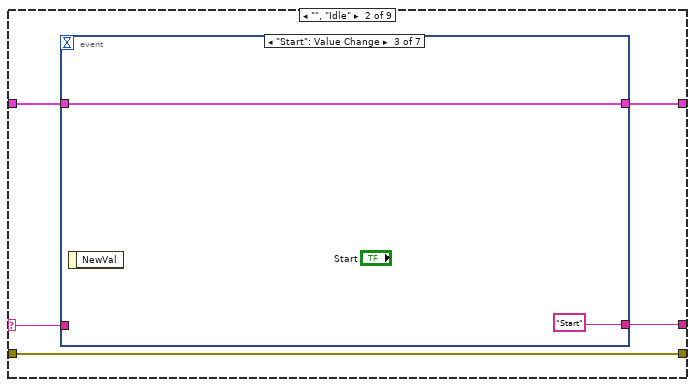
[diagram p3: hidden frame]
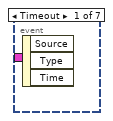
[diagram p4: hidden frame]
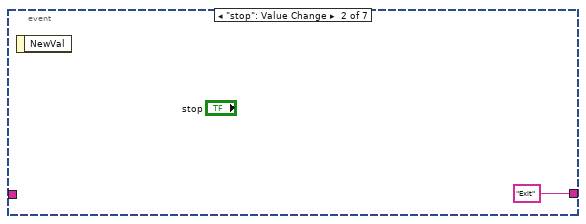
[diagram p5: hidden frame]
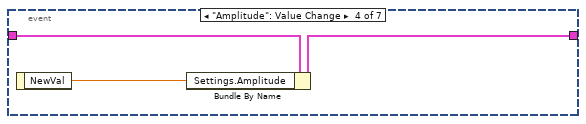
[diagram p6: hidden frame]
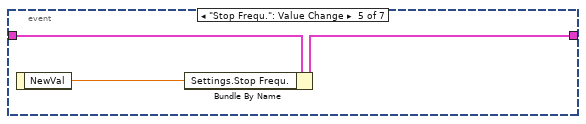
[diagram p7: hidden frame]
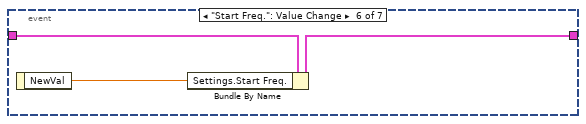
[diagram p8: hidden frame]
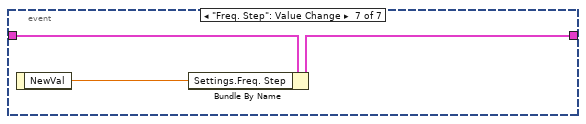
[diagram p9: hidden frame]
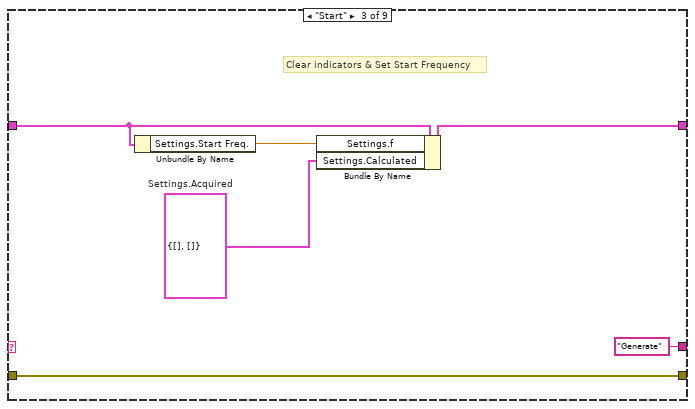
[diagram p10: hidden frame]
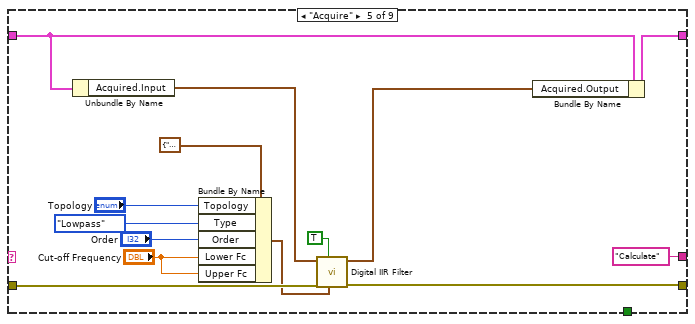
[diagram p11: hidden frame]
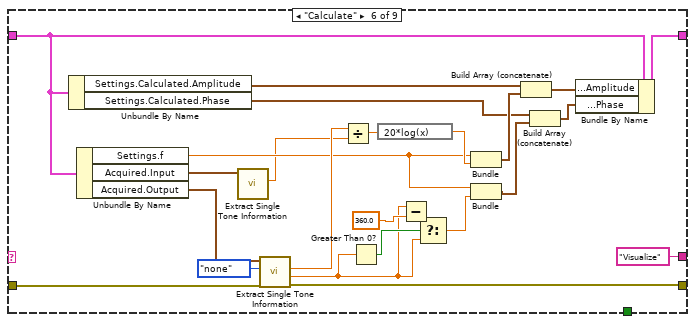
[diagram p12: hidden frame]
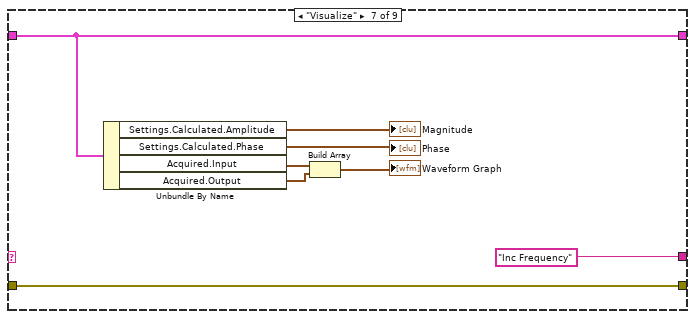
[diagram p13: hidden frame]
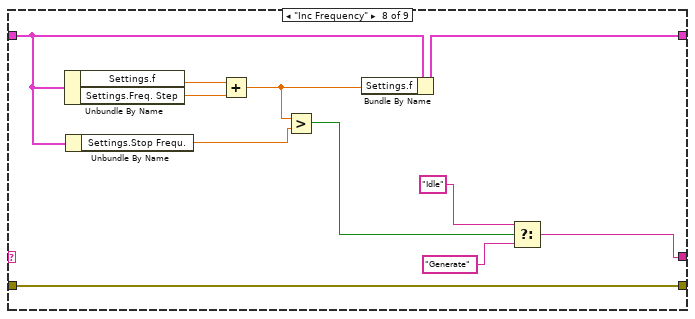
[diagram p14: hidden frame]
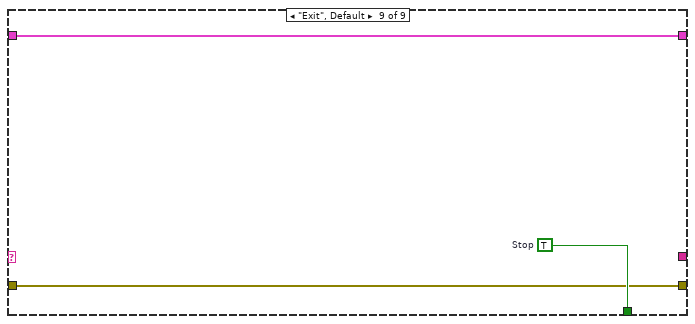
[diagram p15: hidden frame]
diagram:
  w1 = T2 {"Settings"={"f"=0.0, "Start Freq."=0.0, "Freq. Step"=0.0, "Stop Frequ."=0.0, "Amplitude"=0.0, "Calculated"={"Amplitude"=[], "Phase"=[]}}, "Acquired"={"Input"={"t0"=timestamp(0 s since 1904-01-01), "dt"=1.0, "Y"=[]}, "Output"={"t0"=timestamp(0 s since 1904-01-01), "dt"=1.0, "Y"=[]}}}  # Data
  w3 = "Init"  # State
  n1 = while {
    shift-right: [w9] -> _
    shift-left: w3 -> [w11]
    tunnel: errorcluster {"status"=FALSE, "code"=0, "source"=""} ("error constant") -> [w8]
    tunnel: [w7] -> _
    shift-right: [w5] -> _
    shift-left: w1 -> [w6]
    stop <- w10 stop-if-true
    n2 = case shown="\"Generate\"" w11 {
      selector: w11 -> [_ w24 _ _ _ _ _ _ _]
      tunnel: [_ _ _ _ _ _ _ _ w121] -> w10
      tunnel: ["Idle" w23 "Generate" "Acquire" "Calculate" "Visualize" "Inc Frequency" w109 _] -> w9
      tunnel: w8 -> [w13 w22 w41 w60 w75 w82 w104 w108 w119]
      tunnel: [w13 w22 w41 w59 w71 w90 w104 w108 w119] -> w7
      tunnel: w6 -> [w19 w21 w44 w57 w70 w98 w107 w114 w120]
      tunnel: [w18 w20 w45 w56 w69 w99 w107 w116 w120] -> w5
      frame "Init" {
        n3 = Bundle By Name(cluster=w19, "Settings.Amplitude"="Amplitude", "Settings.Freq. Step"="Freq. Step", "Settings.Stop Frequ."="Stop Frequ.", "Settings.Start Freq."="Start Freq.", "Settings.f"="Start Freq.") -> (w18:T2)
      }
      frame "", "Idle" {
        n4 = event shown="[2] \"Start\": Value Change" {
          selector: _ -> [_ _ _ _ _ _ _]
          dyn-events: _ -> [_ _ _ _ _ _ _]
          timeout: _ -> [_ _ _ _ _ _ _]
          tunnel: w24 -> [_ _ _ _ _ _ _]
          tunnel: [_ "Exit" "Start" _ _ _ _] -> w23
          tunnel: w21 -> [_ _ w26 w30 w33 w36 w39]
          tunnel: [_ _ w26 w29 w32 w35 w38] -> w20
          event Timeout {
            n5 = event-data() -> ()  [unwired: 1 in, 3 out]
          }
          event "stop": Value Change {
            n6 = event-data() -> ()  [unwired: 1 in, 1 out]
          }
          event "Start": Value Change {
            n7 = event-data() -> ()  [unwired: 1 in, 1 out]
          }
          event "Amplitude": Value Change {
            n8 = event-data() -> ("NewVal"=w28:dbl)  [unwired: 1 in]
            n9 = Bundle By Name(cluster=w30, "Settings.Amplitude"=w28) -> (w29:T2)
          }
          event "Stop Frequ.": Value Change {
            n10 = event-data() -> ("NewVal"=w31:dbl)  [unwired: 1 in]
            n11 = Bundle By Name(cluster=w33, "Settings.Stop Frequ."=w31) -> (w32:T2)
          }
          event "Start Freq.": Value Change {
            n12 = event-data() -> ("NewVal"=w34:dbl)  [unwired: 1 in]
            n13 = Bundle By Name(cluster=w36, "Settings.Start Freq."=w34) -> (w35:T2)
          }
          event "Freq. Step": Value Change {
            n14 = event-data() -> ("NewVal"=w37:dbl)  [unwired: 1 in]
            n15 = Bundle By Name(cluster=w39, "Settings.Freq. Step"=w37) -> (w38:T2)
          }
        }
      }
      frame "Start" {
        w42 = T6 {"Amplitude"=[], "Phase"=[]}  # Settings.Acquired
        # "Clear indicators & Set Start Frequency"
        n16 = Unbundle By Name(w44) -> ("Settings.Start Freq."=w43:dbl)
        n17 = Bundle By Name(cluster=w44, "Settings.f"=w43, "Settings.Calculated"=w42) -> (w45:T2)
      }
      frame "Generate" {
        # "Generate a stimulus Signal"
        n18 = Unbundle By Name(w57) -> ("Settings.Amplitude"=w58:dbl)
        n19 = Unbundle By Name(w57) -> ("Settings.f"=w53:dbl)
        n20 = Reciprocal(x=w53) -> (1/x=w51:dbl)
        n21 = Multiply(x=w53, y=100.0) -> (x*y=w50:dbl)
        n22 = Multiply(x=w51, y=10.0) -> (x*y=w47:dbl)
        n23 = Multiply(x=w47, y=w50) -> (x*y=w49:dbl)
        n24 = Bundle By Name(cluster=cluster{"Fs":dbl, "Count":dbl} {"Fs"=1000.0, "Count"=1000.0} ("sampling info"), "Fs"=w50, "Count"=w49) -> (w54:cluster{"Fs":dbl, "Count":dbl})
        n25 = call <vilib>:"Sine Waveform.vi"("sampling info"=w54, "error in (no error)"=w60, "amplitude"=w58, "frequency"=w53) -> ("error out"=w59:errorcluster, "signal out"=w48:waveform(dbl))  [unwired: 6 in]
        n26 = Bundle By Name(cluster=w57, "Acquired.Input"=w48) -> (w56:T2)
      }
      frame "Acquire" {
        n27 = Unbundle By Name(w70) -> ("Acquired.Input"=w72:waveform(dbl))
        n28 = Bundle By Name(cluster=T4 {"Topology"=enum."Butterworth", "Type"=enum."Lowpass", "Order"=1, "Lower Fc"=10000.0, "Upper Fc"=10000.0, "PB Ripple"=1.0, "SB Attenuation"=60.0} ("IIR filter specifications"), "Topology"="Topology", "Type"=T3."Lowpass", "Order"="Order", "Lower Fc"="Cut-off Frequency", "Upper Fc"="Cut-off Frequency") -> (w67:T4)
        n29 = call-poly <vilib>:"Digital IIR Filter.vi"("IIR filter specifications"=w67, "reset filter"=TRUE, "error in (no error)"=w75, "signal in"=w72) -> ("error out"=w71:errorcluster, "signal out"=w68:waveform(dbl))  [unwired: 5 in, 1 out]
        n30 = Bundle By Name(cluster=w70, "Acquired.Output"=w68) -> (w69:T2)
      }
      frame "Calculate" {
        n31 = Unbundle By Name(w98) -> ("Settings.Calculated.Amplitude"=w97:cluster{"X":dbl, "Y":dbl}[], "Settings.Calculated.Phase"=w87:cluster{"X":dbl, "Y":dbl}[])
        n32 = Unbundle By Name(w98) -> ("Settings.f"=w88:dbl, "Acquired.Input"=w91:waveform(dbl), "Acquired.Output"=w83:waveform(dbl))
        n33 = call-poly <vilib>:"Extract Single Tone Information.vi"("time signal in"=w91) -> ("detected amplitude"=w84:dbl)  [unwired: 5 in, 5 out]
        n34 = call-poly <vilib>:"Extract Single Tone Information.vi"("error in (no error)"=w82, "export mode"=T5."none", "time signal in"=w83) -> ("error out"=w90:errorcluster, "detected phase (deg)"=w77:dbl, "detected amplitude"=w89:dbl)  [unwired: 3 in, 3 out]
        n35 = Divide(x=w89, y=w84) -> (x/y=w94:dbl)
        n36 = Greater Than 0?(x=w77) -> (x > 0?=w79:bool)
        n37 = expression code="20*log(x)"(w94) -> (w92:dbl)
        n38 = Subtract(x=w77, y=360.0) -> (x-y=w78:dbl)
        n39 = Select(t=w78, s=w79, f=w77) -> (s? t:f=w76:dbl)
        n40 = Bundle("f"=w88, w92) -> (w93:cluster{"f":dbl, dbl})  [unwired: 1 in]
        n41 = Bundle("f"=w88, "detected phase (deg)"=w76) -> (w85:cluster{"f":dbl, "detected phase (deg)":dbl})  [unwired: 1 in]
        n42 = Build Array (concatenate)(w97, w93) -> (w96:cluster{"f":dbl, "Y":dbl}[])
        n43 = Build Array (concatenate)(w87, w85) -> (w86:cluster{"f":dbl, "detected phase (deg)":dbl}[])
        n44 = Bundle By Name(cluster=w98, "Settings.Calculated.Amplitude"=w96, "Settings.Calculated.Phase"=w86) -> (w99:T2)
      }
      frame "Visualize" {
        n45 = Unbundle By Name(w107) -> ("Settings.Calculated.Amplitude"=→"Magnitude":cluster{"X":dbl, "Y":dbl}[], "Settings.Calculated.Phase"=→"Phase":cluster{"X":dbl, "Y":dbl}[], "Acquired.Input"=w102:waveform(dbl), "Acquired.Output"=w101:waveform(dbl))
        n46 = Build Array(w102, w101) -> (→"Waveform Graph":waveform(dbl)[])
      }
      frame "Inc Frequency" {
        n47 = Unbundle By Name(w114) -> ("Settings.f"=w118:dbl, "Settings.Freq. Step"=w117:dbl)
        n48 = Unbundle By Name(w114) -> ("Settings.Stop Frequ."=w113:dbl)
        n49 = Add(x=w118, y=w117) -> (x+y=w115:dbl)
        n50 = Greater?(x=w115, y=w113) -> (0:w112:bool)
        n51 = Bundle By Name(cluster=w114, "Settings.f"=w115) -> (w116:T2)
        n52 = Select(t="Idle", s=w112, f="Generate") -> (s? t:f=w109:string)
      }
      frame "Exit", Default {
        w121 = TRUE  # Stop
      }
    }
    n53 = Wait (ms)(milliseconds to wait="Timing (ms)") -> ()  [unwired: 1 out]
  }
